vi "torreHanoi.vi"() -> ()   [LabVIEW 2020]
uses:
  <vilib>/Analysis/Matrix/Datatypes/RealMatrix.ctl
  <vilib>/Utility/miscctls.llb/LVPositionTypeDef.ctl
  <vilib>/Utility/miscctls.llb/LVBoundsTypeDef.ctl
  <vilib>/Analysis/Matrix/NI_Matrix.lvlib
panel:
  out "PosAntPiezaCuatro":T1
  out "PosAntPiezaCinco":T1
  out "PosAntPiezaTres":T1
  out "PosAntPiezaDos":T1
  out "Posicion":i32
  out "Torre":i8
  out "posPiezaDos":i32[][](array[numeric])
  out "posPiezaTres":i32[][](array[numeric])
  out "posPiezaUno":i32[][](array[numeric])
  out "posPiezaCinco":i32[](array[numeric])
  out "posPiezaCuatro":i32[][](array[numeric])
  out "estadoTorreTres":i32[](array[numeric])
  out "estadoTorreUno":i32[](array[numeric])
  out "estadoTorreDos":i32[](array[numeric])
  out "PosAntPiezaUno":T1
  out "¿Pieza?":i8
  out "matrizPosIniciales":T2
  out "numMov":dbl
  out "minMov":dbl
  in  "numPiezas":enum16{"5", "4", "3"}(ring)
  in  "Iniciar":bool
  out "PiezaCinco":bool
  out "PiezaCuatro":bool
  out "PiezaTres":bool
  out "PiezaDos":bool
  in  "Deterner":bool
  out "PiezaUno":bool
  out "TorreUno":u8(slide) scale=0.0..100.0
  out "TorreDos":u8(slide) scale=0.0..100.0
  out "TorreTres":u8(slide) scale=0.0..100.0
  # "Número de Piezas"
  # "Minimo de Movimientos"
  # "Tus Movimientos"
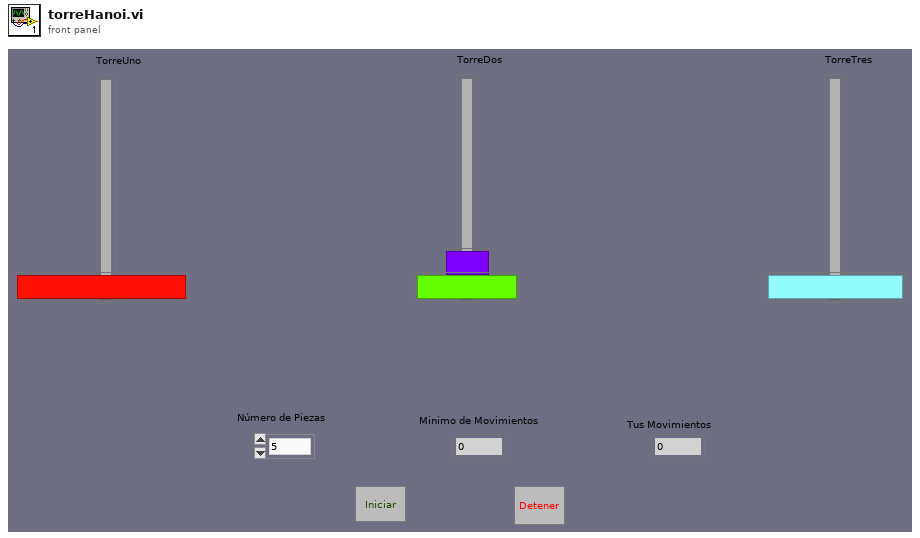
[diagram p1: front panel]
types:
  T1 = typedef "LVPositionTypeDef.ctl" = cluster{"Left":i32, "Top":i32}
  T2 = typedef "NI_Matrix.lvlib/RealMatrix.ctl" = dbl[][]
  T3 = typedef "LVBoundsTypeDef.ctl" = cluster{"Width":u32, "Height":u32}
  T4 = typedef "LVPoint32TypeDef.ctl" = cluster{"Horizontal":i32, "Vertical":i32}
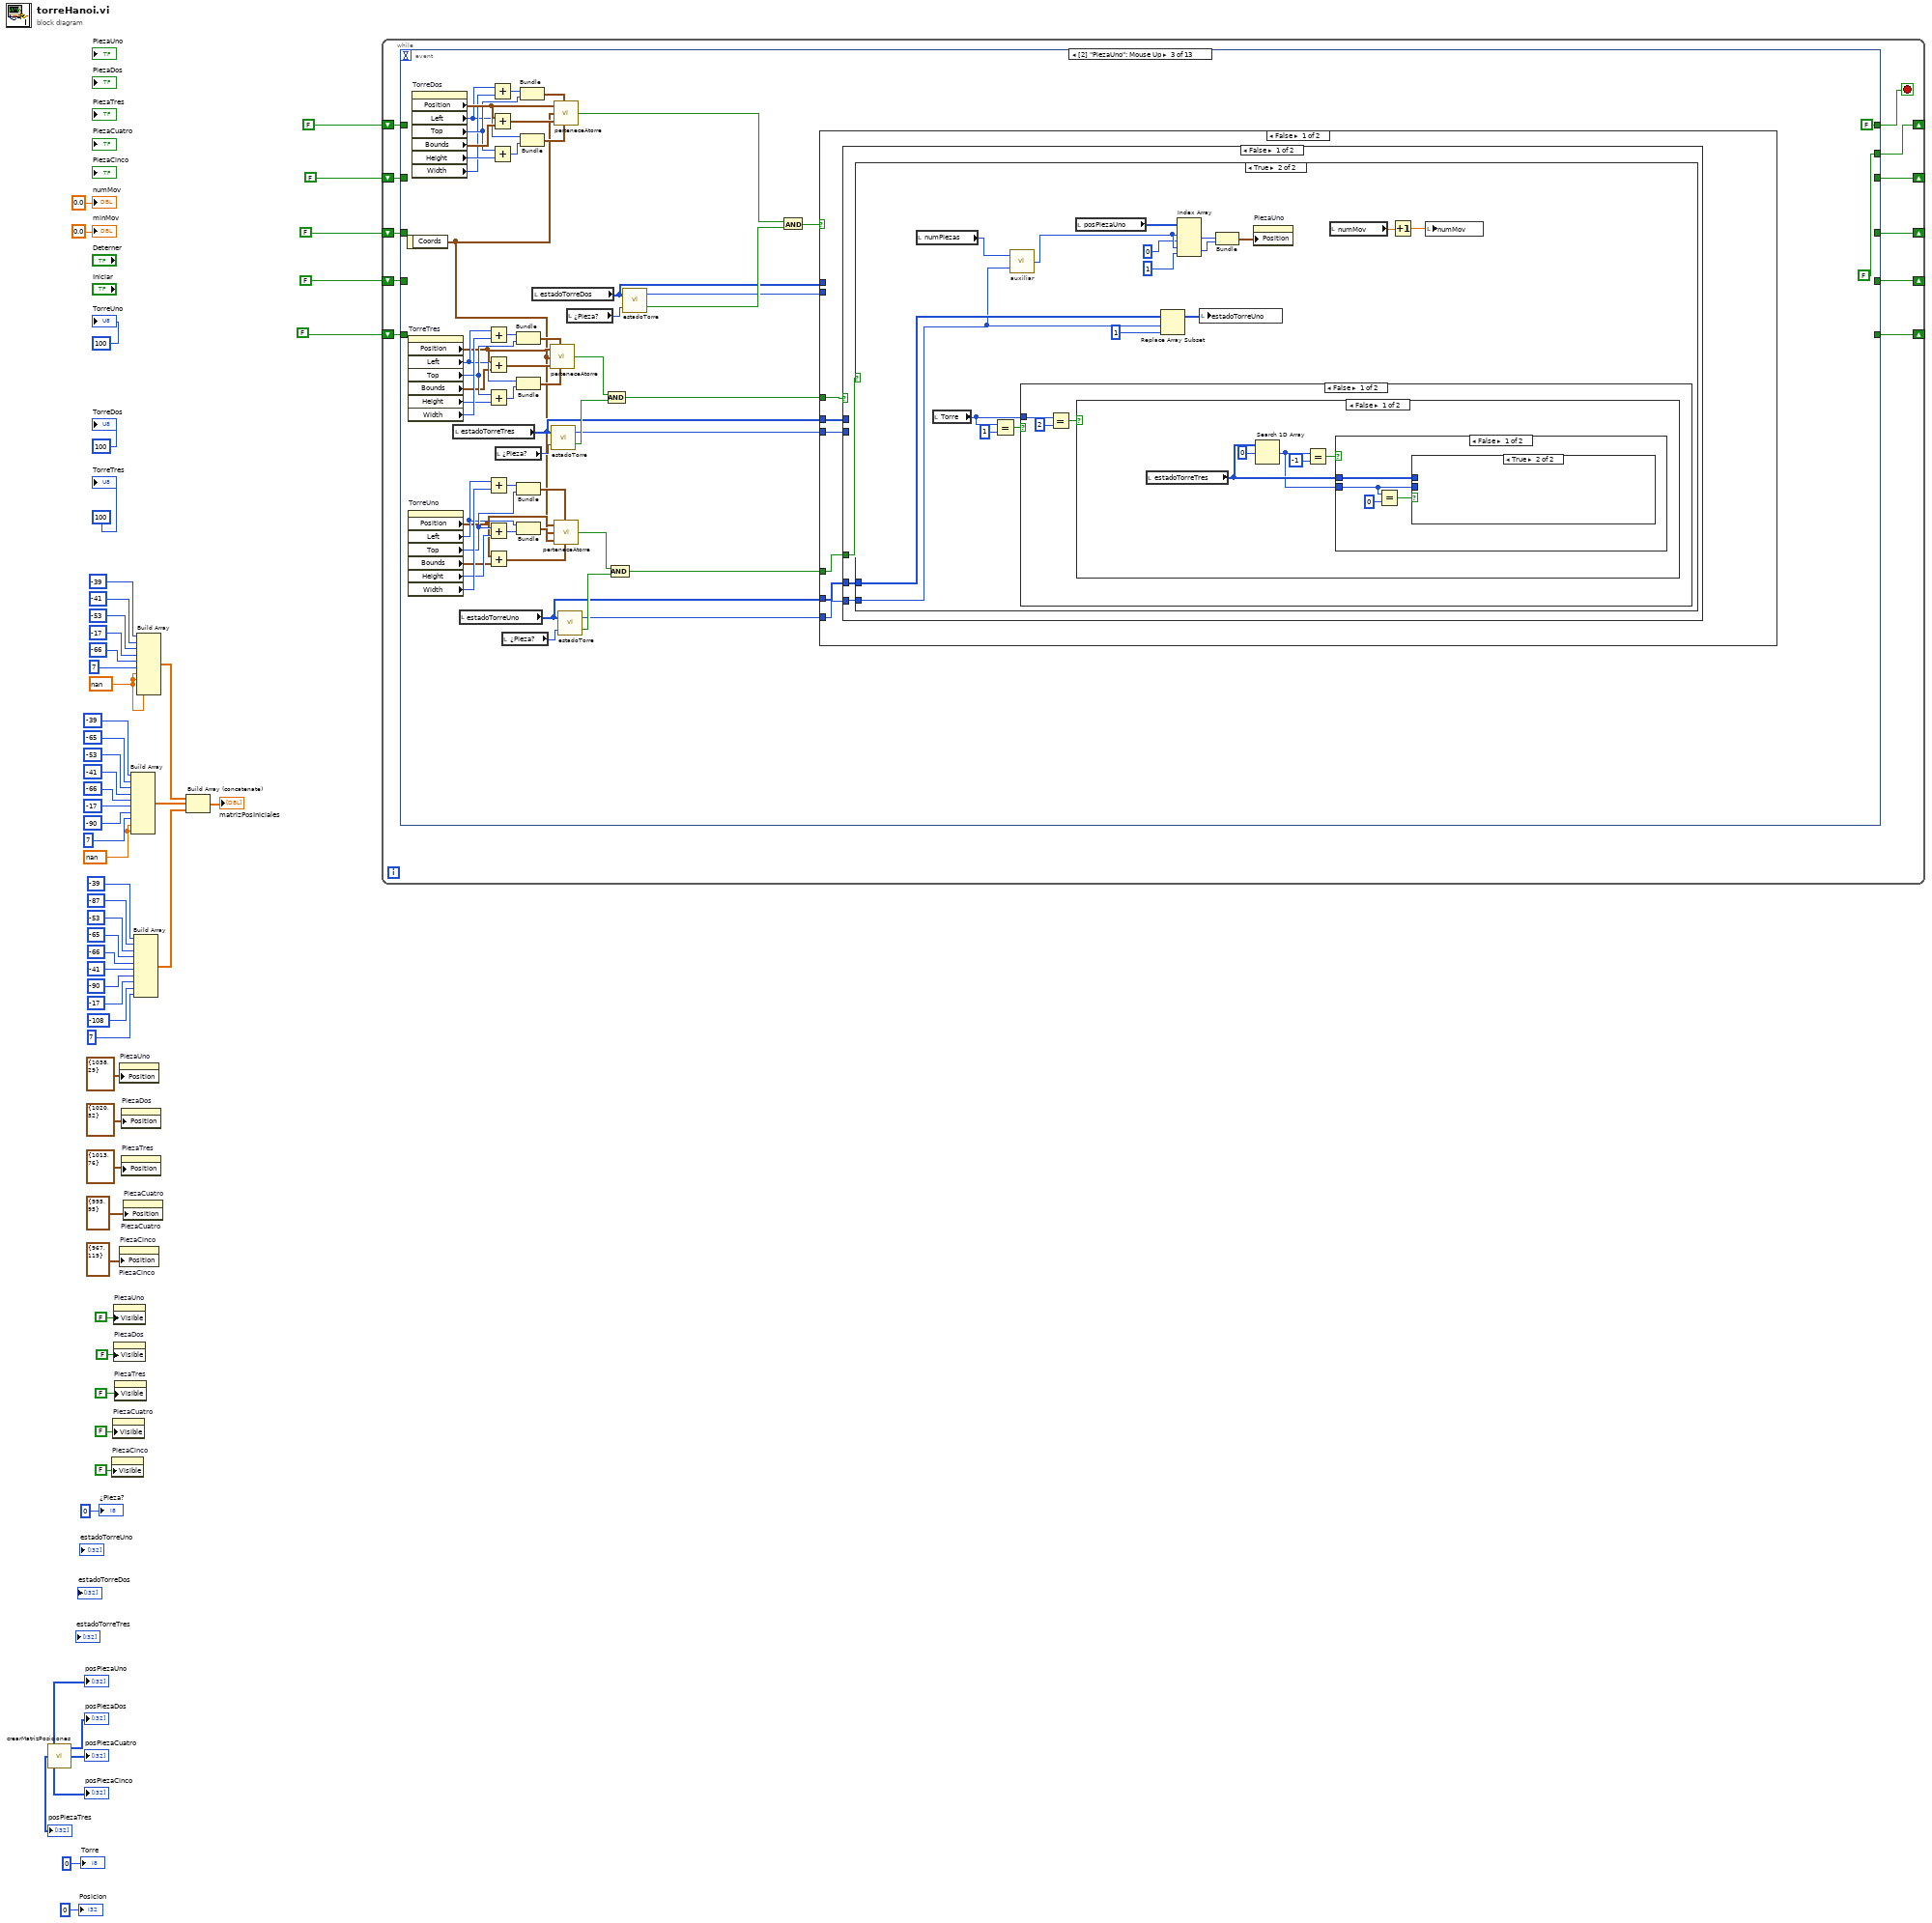
[diagram p0: block diagram]
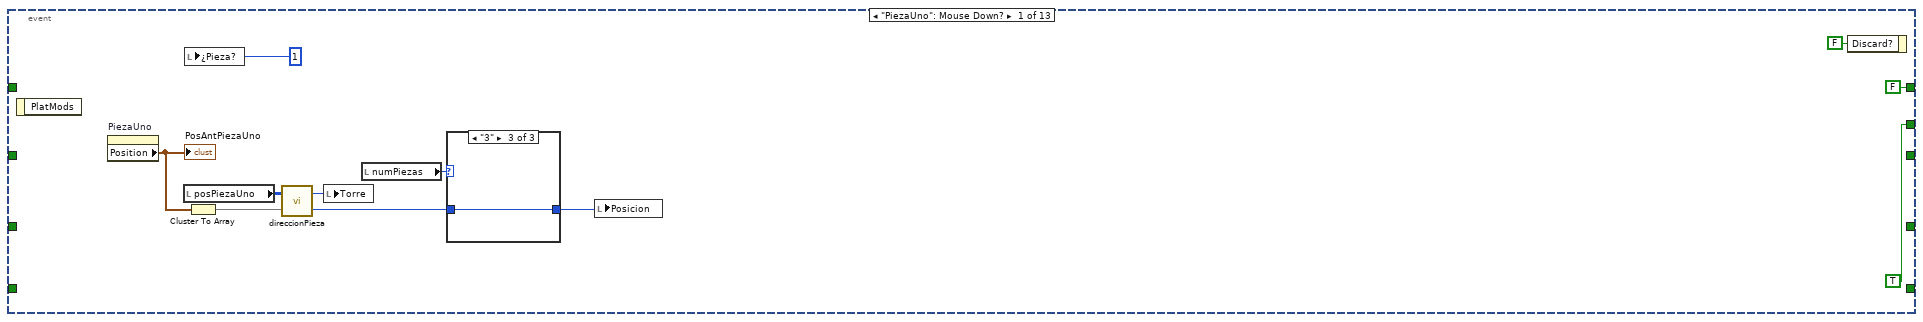
[diagram p2: hidden frame]
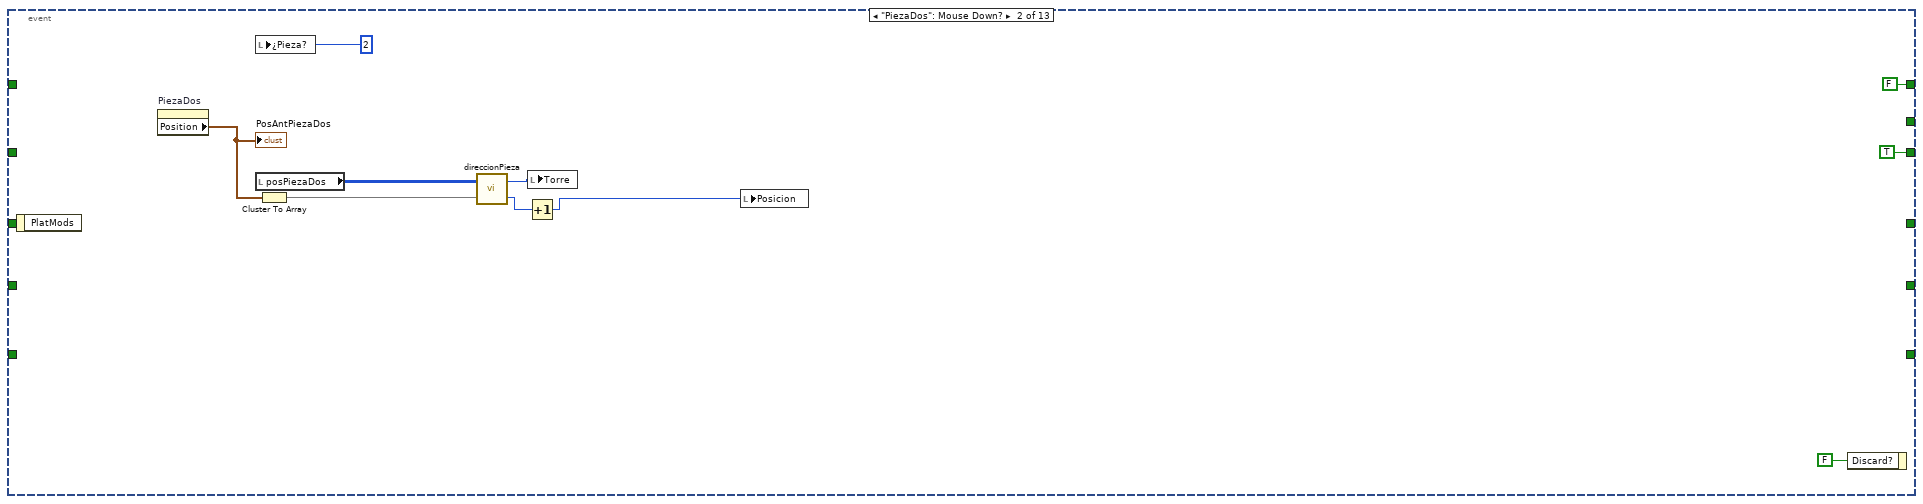
[diagram p5: hidden frame]
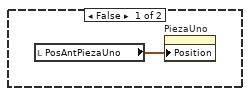
[diagram p6: hidden frame]
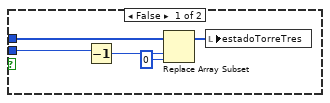
[diagram p7: hidden frame]
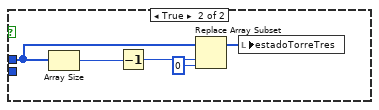
[diagram p8: hidden frame]
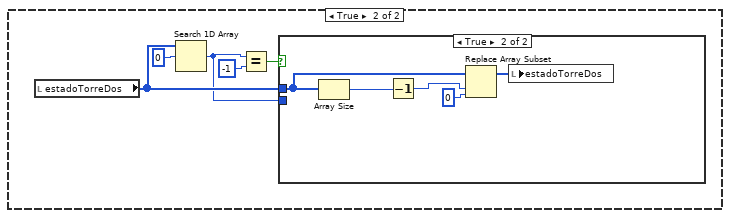
[diagram p9: hidden frame]
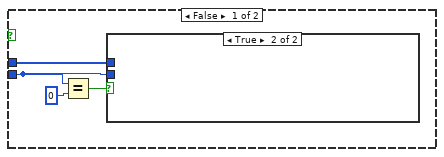
[diagram p10: hidden frame]
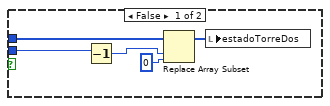
[diagram p11: hidden frame]
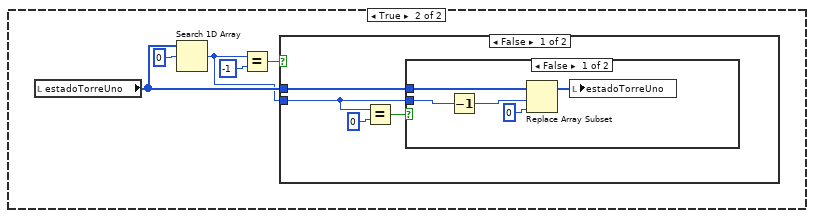
[diagram p12: hidden frame]
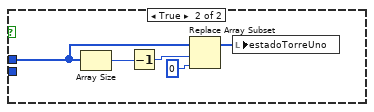
[diagram p14: hidden frame]
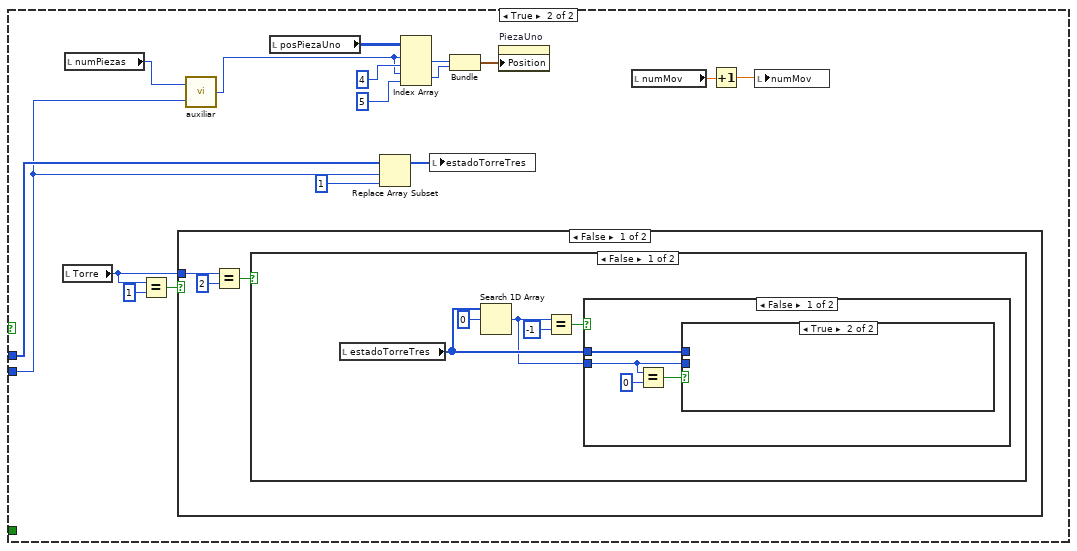
[diagram p15: hidden frame]
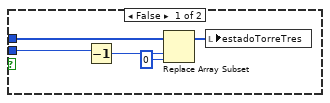
[diagram p16: hidden frame]
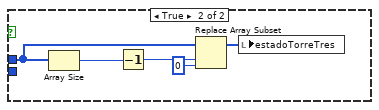
[diagram p17: hidden frame]
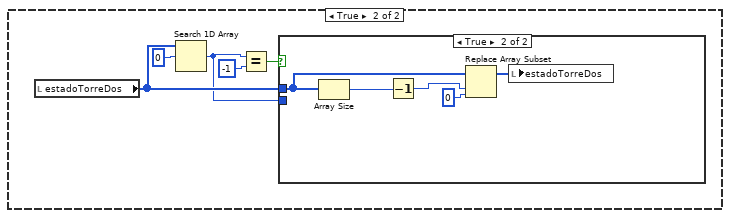
[diagram p18: hidden frame]
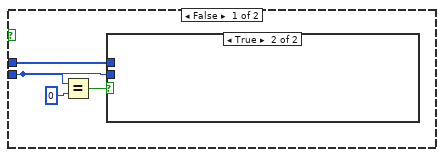
[diagram p19: hidden frame]
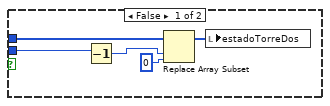
[diagram p20: hidden frame]
diagram:
  w42 = nan
  w51 = nan
  n1 = call "crearMatrizPosiciones.vi"() -> ("posPiezaCuatro"=→"posPiezaCuatro":i32[][], "posPiezaDos"=→"posPiezaDos":i32[][], "posPiezaCinco"=→"posPiezaCinco":i32[], "posPiezaTres"=→"posPiezaTres":i32[][], "posPiezaUno"=→"posPiezaUno":i32[][])  [unwired: 1 in]
  n2 = property on="PiezaCinco" class="Bool (strict)"("Visible"=FALSE ("PiezaCinco")) -> ()  [unwired: 2 in, 2 out]
  n3 = property on="PiezaCuatro" class="Bool (strict)"("Visible"=FALSE ("PiezaCuatro")) -> ()  [unwired: 2 in, 2 out]
  n4 = property on="PiezaUno" class="Bool (strict)"("Visible"=FALSE) -> ()  [unwired: 2 in, 2 out]
  n5 = property on="PiezaDos" class="Bool (strict)"("Visible"=FALSE ("PiezaDos")) -> ()  [unwired: 2 in, 2 out]
  n6 = property on="PiezaTres" class="Bool (strict)"("Visible"=FALSE) -> ()  [unwired: 2 in, 2 out]
  n7 = property on="PiezaUno" class="Bool (strict)"("Position"=T1 {"Left"=1038, "Top"=29}) -> ()  [unwired: 2 in, 2 out]
  n8 = property on="PiezaCinco" class="Bool (strict)"("Position"=T1 {"Left"=967, "Top"=119}) -> ()  [unwired: 2 in, 2 out]
  n9 = property on="PiezaCinco" class="Bool (strict)"("Position"=T1 {"Left"=967, "Top"=119}) -> ()  [unwired: 2 in, 2 out]
  n10 = property on="PiezaDos" class="Bool (strict)"("Position"=T1 {"Left"=1020, "Top"=52}) -> ()  [unwired: 2 in, 2 out]
  n11 = property on="PiezaTres" class="Bool (strict)"("Position"=T1 {"Left"=1013, "Top"=76}) -> ()  [unwired: 2 in, 2 out]
  n12 = property on="PiezaCuatro" class="Bool (strict)"("Position"=T1 {"Left"=995, "Top"=95}) -> ()  [unwired: 2 in, 2 out]
  n13 = property on="PiezaCuatro" class="Bool (strict)"("Position"=T1 {"Left"=995, "Top"=95}) -> ()  [unwired: 2 in, 2 out]
  n14 = Build Array(-39, -65 ("element"), -53 ("element"), -41 ("element"), -66 ("element"), -17 ("element"), -90 ("element"), 7 ("element"), w42, w42) -> (w30:T2)
  n15 = Build Array(-39, -87 ("element"), -53 ("element"), -65 ("element"), -66 ("element"), -41 ("element"), -90 ("element"), -17 ("element"), -108 ("element"), 7 ("element")) -> (w29:T2)
  n16 = Build Array(-39, -41 ("element"), -53 ("element"), -17 ("element"), -66 ("element"), 7 ("element"), w51, w51, w51, w51) -> (w31:T2)
  n17 = Build Array (concatenate)(w31, w30, w29) -> (→"matrizPosIniciales":T2)
  n18 = while {
    shift-right: [w70] -> _
    shift-left: FALSE -> [w69]
    shift-right: [w68] -> _
    shift-left: FALSE -> [w67]
    shift-right: [w66] -> _
    shift-left: FALSE -> [w65]
    shift-right: [w63] -> _
    shift-left: FALSE -> [w64]
    shift-right: [w62] -> _
    shift-left: FALSE -> [w61]
    stop <- w71 stop-if-true
    n19 = event shown="[2] \"PiezaUno\": Mouse Up" {
      selector: _ -> [_ _ _ _ _ _ _ _ _ _ _ _ _]
      dyn-events: _ -> [_ _ _ _ _ _ _ _ _ _ _ _ _]
      timeout: _ -> [_ _ _ _ _ _ _ _ _ _ _ _ _]
      tunnel: [FALSE FALSE FALSE FALSE FALSE TRUE _ FALSE FALSE FALSE FALSE FALSE _] -> w71
      tunnel: [TRUE _ FALSE w397 _ _ _ _ _ _ _ _ _] -> w70
      tunnel: w69 -> [_ _ _ w397 _ _ _ _ _ _ _ _ _]
      tunnel: [_ TRUE _ w395 _ _ _ FALSE _ _ _ _ _] -> w68
      tunnel: w67 -> [_ _ _ w395 _ _ _ _ _ _ _ _ _]
      tunnel: [_ _ _ w394 _ _ _ _ TRUE FALSE _ _ _] -> w66
      tunnel: w65 -> [_ _ _ w394 _ _ _ _ _ _ _ _ _]
      tunnel: w64 -> [_ _ _ w391 _ _ _ _ _ _ _ _ _]
      tunnel: [_ _ _ w391 FALSE _ _ _ _ _ TRUE _ _] -> w63
      tunnel: [_ _ _ w392 _ _ _ _ _ _ _ TRUE _] -> w62
      tunnel: w61 -> [_ _ _ w392 _ _ _ _ _ _ _ _ _]
      event "PiezaUno": Mouse Down? {
        n20 = event-data() -> ()  [unwired: 1 in, 1 out]
        n21 = property on="PiezaUno" class="Bool (strict)"() -> ("Position"=w78:T1)  [unwired: 2 in, 2 out]
        "PosAntPiezaUno" <- w78
        n22 = local read "posPiezaUno"() -> (w76:i32[][])
        n23 = local write "¿Pieza?"(i8 1 ("¿Pieza?")) -> ()
        n24 = Cluster To Array(cluster=w78) -> (array=w77:i32[])
        n25 = call "direccionPieza.vi"("posicion"=w77, "matrizPosiciones"=w76) -> ("Posicion"=w72:i32, "Torre"=w75:i8)
        n26 = local write "Torre"(w75) -> ()
        n27 = local read "numPiezas"() -> (w74:enum16{"5", "4", "3"})
        n28 = case shown="\"3\"" w74 {
          tunnel: [w83 w84 w85] -> w73
          tunnel: w72 -> [w83 w84 w85]
          frame "5", Default {
          }
          frame "4" {
          }
          frame "3" {
          }
        }
        n29 = local write "Posicion"(w73) -> ()
        n30 = event-data("Discard?"=FALSE) -> ()  [unwired: 1 in, 1 out]
      }
      event "PiezaDos": Mouse Down? {
        n31 = event-data() -> ()  [unwired: 1 in, 1 out]
        n32 = property on="PiezaDos" class="Bool (strict)"() -> ("Position"=w91:T1)  [unwired: 2 in, 2 out]
        "PosAntPiezaDos" <- w91
        n33 = local write "¿Pieza?"(i8 2 ("¿Pieza?")) -> ()
        n34 = local read "posPiezaDos"() -> (w93:i32[][])
        n35 = Cluster To Array(cluster=w91) -> (array=w94:i32[])
        n36 = call "direccionPieza.vi"("posicion"=w94, "matrizPosiciones"=w93) -> ("Posicion"=w87:i32, "Torre"=w92:i8)
        n37 = Increment(x=w87) -> (x+1=w86:i32)
        n38 = local write "Torre"(w92) -> ()
        n39 = local write "Posicion"(w86) -> ()
        n40 = event-data("Discard?"=FALSE) -> ()  [unwired: 1 in, 1 out]
      }
      event "PiezaUno": Mouse Up {
        n41 = event-data() -> ("Coords"=w102:T4)  [unwired: 1 in]
        n42 = property on="TorreTres" class="Slide (strict)"() -> ("Position"=w121:T1, "Left"=w124:i32, "Top"=w127:i32, "Bounds"=w122:T3, "Height"=w126:u32, "Width"=w130:u32)  [unwired: 2 in, 2 out]
        n43 = property on="TorreUno" class="Slide (strict)"() -> ("Position"=w105:T1, "Left"=w107:i32, "Top"=w110:i32, "Bounds"=w104:T3, "Height"=w109:u32, "Width"=w113:u32)  [unwired: 2 in, 2 out]
        n44 = property on="TorreDos" class="Slide (strict)"() -> ("Position"=w144:T1, "Left"=w139:i32, "Top"=w142:i32, "Bounds"=w145:T3, "Height"=w141:u32, "Width"=w140:u32)  [unwired: 2 in, 2 out]
        n45 = local read "estadoTorreTres"() -> (w115:i32[])
        n46 = local read "estadoTorreUno"() -> (w96:i32[])
        n47 = Add(x=w124, y=w130) -> (x+y=w129:u32)
        n48 = Add(x=w121, y=w122) -> (x+y=w120:T3)
        n49 = Add(x=w127, y=w126) -> (x+y=w125:u32)
        n50 = Add(x=w107, y=w113) -> (x+y=w111:u32)
        n51 = Add(x=w110, y=w109) -> (x+y=w108:u32)
        n52 = Add(x=w105, y=w104) -> (x+y=w103:T3)
        n53 = Add(x=w139, y=w140) -> (x+y=w147:u32)
        n54 = Add(x=w144, y=w145) -> (x+y=w143:T3)
        n55 = Add(x=w142, y=w141) -> (x+y=w138:u32)
        n56 = local read "¿Pieza?"() -> (w119:i8)
        n57 = local read "¿Pieza?"() -> (w101:i8)
        n58 = Bundle(w129, "Top"=w127) -> (w128:cluster{u32, "Top":i32})  [unwired: 1 in]
        n59 = Bundle("Left"=w124, w125) -> (w123:cluster{"Left":i32, u32})  [unwired: 1 in]
        n60 = Bundle(w111, "Top"=w110) -> (w112:cluster{u32, "Top":i32})  [unwired: 1 in]
        n61 = Bundle("Left"=w107, w108) -> (w106:cluster{"Left":i32, u32})  [unwired: 1 in]
        n62 = Bundle(w147, "Top"=w142) -> (w146:cluster{u32, "Top":i32})  [unwired: 1 in]
        n63 = Bundle("Left"=w139, w138) -> (w137:cluster{"Left":i32, u32})  [unwired: 1 in]
        n64 = local read "estadoTorreDos"() -> (w131:i32[])
        n65 = call "perteneceAtorre.vi"("P1"=w121, "P2"=w128, "P"=w102, "P3"=w120, "P4"=w123) -> ("out"=w118:bool)
        n66 = call "estadoTorre.vi"("¿pieza?"=w119, "estadoTorre"=w115) -> ("¿disponible?"=w117:bool, "posicionCero"=w116:i32)
        n67 = call "perteneceAtorre.vi"("P1"=w144, "P2"=w146, "P"=w102, "P3"=w143, "P4"=w137) -> ("out"=w135:bool)
        n68 = call "perteneceAtorre.vi"("P1"=w105, "P2"=w112, "P"=w102, "P3"=w106, "P4"=w103) -> ("out"=w100:bool)
        n69 = call "estadoTorre.vi"("¿pieza?"=w101, "estadoTorre"=w96) -> ("¿disponible?"=w99:bool, "posicionCero"=w97:i32)
        n70 = local read "¿Pieza?"() -> (w134:i8)
        n71 = And(x=w118, y=w117) -> (x .and. y?=w114:bool)
        n72 = And(x=w100, y=w99) -> (x .and. y?=w98:bool)
        n73 = call "estadoTorre.vi"("¿pieza?"=w134, "estadoTorre"=w131) -> ("¿disponible?"=w133:bool, "posicionCero"=w132:i32)
        n74 = And(x=w135, y=w133) -> (x .and. y?=w136:bool)
        n75 = case shown="False" w136 {
          tunnel: w132 -> [_ w320]
          tunnel: w131 -> [_ w324]
          tunnel: w116 -> [w153 _]
          tunnel: w115 -> [w154 _]
          tunnel: w114 -> [w155 _]
          tunnel: w98 -> [w152 _]
          tunnel: w97 -> [w150 _]
          tunnel: w96 -> [w151 _]
          frame False {
            n76 = case shown="False" w155 {
              tunnel: w154 -> [_ w243]
              tunnel: w153 -> [_ w242]
              tunnel: w152 -> [w158 _]
              tunnel: w151 -> [w157 _]
              tunnel: w150 -> [w156 _]
              frame False {
                n77 = case shown="True" w158 {
                  tunnel: w157 -> [_ w166]
                  tunnel: w156 -> [_ w165]
                  frame False {
                    n78 = local read "PosAntPiezaUno"() -> (w159:T1)
                    n79 = property on="PiezaUno" class="Bool (strict)"("Position"=w159) -> ()  [unwired: 2 in, 2 out]
                  }
                  frame True {
                    n80 = local read "numPiezas"() -> (w171:enum16{"5", "4", "3"})
                    n81 = local read "Torre"() -> (w160:i8)
                    n82 = Equal?(x=w160, y=i8 1) -> (x = y?=w162:bool)
                    n83 = call "auxiliar.vi"("posicion"=w165, "numPiezas"=w171) -> ("posicion"=w170:i32)
                    n84 = case shown="False" w162 {
                      tunnel: w160 -> [w177 _]
                      frame False {
                        n85 = Equal?(x=w177, y=i8 2) -> (x = y?=w178:bool)
                        n86 = case shown="False" w178 {
                          frame False {
                            n87 = local read "estadoTorreTres"() -> (w183:i32[])
                            n88 = Search 1D Array(1D array=w183, element=0) -> (index of element=w182:i32)  [unwired: 1 in]
                            n89 = Equal?(x=w182, y=-1) -> (x = y?=w184:bool)
                            n90 = case shown="False" w184 {
                              tunnel: w183 -> [w185 w196]
                              tunnel: w182 -> [w186 _]
                              frame False {
                                n91 = Equal?(x=w186, y=0) -> (x = y?=w187:bool)
                                n92 = case shown="True" w187 {
                                tunnel: w186 -> [w193 _]
                                tunnel: w185 -> [w191 _]
                                frame False {
                                n93 = Decrement(x=w193) -> (x-1=w192:i32)
                                n94 = Replace Array Subset(array=w191, new element=0 ("new element/subarray"), index=w192) -> (w189:i32[])
                                n95 = local write "estadoTorreTres"(w189) -> ()
                                }
                                frame True {
                                }
                                }
                              }
                              frame True {
                                n96 = Array Size(array=w196) -> (size(s)=w198:i32)
                                n97 = Decrement(x=w198) -> (x-1=w197:i32)
                                n98 = Replace Array Subset(array=w196, new element=0 ("new element/subarray"), index=w197) -> (w194:i32[])
                                n99 = local write "estadoTorreTres"(w194) -> ()
                              }
                            }
                          }
                          frame True {
                            n100 = local read "estadoTorreDos"() -> (w200:i32[])
                            n101 = Search 1D Array(1D array=w200, element=0) -> (index of element=w199:i32)  [unwired: 1 in]
                            n102 = Equal?(x=w199, y=-1) -> (x = y?=w201:bool)
                            n103 = case shown="True" w201 {
                              tunnel: w200 -> [w204 w215]
                              tunnel: w199 -> [w205 _]
                              frame False {
                                n104 = Equal?(x=w205, y=0) -> (x = y?=w206:bool)
                                n105 = case shown="True" w206 {
                                tunnel: w205 -> [w212 _]
                                tunnel: w204 -> [w210 _]
                                frame False {
                                n106 = Decrement(x=w212) -> (x-1=w211:i32)
                                n107 = Replace Array Subset(array=w210, new element=0 ("new element/subarray"), index=w211) -> (w208:i32[])
                                n108 = local write "estadoTorreDos"(w208) -> ()
                                }
                                frame True {
                                }
                                }
                              }
                              frame True {
                                n109 = Array Size(array=w215) -> (size(s)=w217:i32)
                                n110 = Decrement(x=w217) -> (x-1=w216:i32)
                                n111 = Replace Array Subset(array=w215, new element=0 ("new element/subarray"), index=w216) -> (w213:i32[])
                                n112 = local write "estadoTorreDos"(w213) -> ()
                              }
                            }
                          }
                        }
                      }
                      frame True {
                        n113 = local read "estadoTorreUno"() -> (w219:i32[])
                        n114 = Search 1D Array(1D array=w219, element=0) -> (index of element=w218:i32)  [unwired: 1 in]
                        n115 = Equal?(x=w218, y=-1) -> (x = y?=w220:bool)
                        n116 = case shown="False" w220 {
                          tunnel: w219 -> [w223 w234]
                          tunnel: w218 -> [w224 _]
                          frame False {
                            n117 = Equal?(x=w224, y=0) -> (x = y?=w225:bool)
                            n118 = case shown="False" w225 {
                              tunnel: w224 -> [w231 _]
                              tunnel: w223 -> [w229 _]
                              frame False {
                                n119 = Decrement(x=w231) -> (x-1=w230:i32)
                                n120 = Replace Array Subset(array=w229, new element=0 ("new element/subarray"), index=w230) -> (w227:i32[])
                                n121 = local write "estadoTorreUno"(w227) -> ()
                              }
                              frame True {
                              }
                            }
                          }
                          frame True {
                            n122 = Array Size(array=w234) -> (size(s)=w236:i32)
                            n123 = Decrement(x=w236) -> (x-1=w235:i32)
                            n124 = Replace Array Subset(array=w234, new element=0 ("new element/subarray"), index=w235) -> (w232:i32[])
                            n125 = local write "estadoTorreUno"(w232) -> ()
                          }
                        }
                      }
                    }
                    n126 = local read "posPiezaUno"() -> (w175:i32[][])
                    n127 = Replace Array Subset(array=w166, new element=1, index=w165) -> (w176:i32[])
                    n128 = Index Array(array=w175, index (row) #1=w170, index (col) #1=0 ("disabled index (col)"), index (row) #2=w170, index (col) #2=1 ("disabled index (col)")) -> (element #1=w174:i32, element #2=w172:i32)
                    n129 = local write "estadoTorreUno"(w176) -> ()
                    n130 = Bundle(w174, w172) -> (w173:cluster{i32, i32})  [unwired: 1 in]
                    n131 = property on="PiezaUno" class="Bool (strict)"("Position"=w173) -> ()  [unwired: 2 in, 2 out]
                    n132 = local read "numMov"() -> (w164:dbl)
                    n133 = Increment(x=w164) -> (x+1=w163:dbl)
                    n134 = local write "numMov"(w163) -> ()
                  }
                }
              }
              frame True {
                n135 = local read "Torre"() -> (w238:i8)
                n136 = local read "numPiezas"() -> (w245:enum16{"5", "4", "3"})
                n137 = Equal?(x=w238, y=i8 1) -> (x = y?=w239:bool)
                n138 = case shown="False" w239 {
                  tunnel: w238 -> [w254 _]
                  frame False {
                    n139 = Equal?(x=w254, y=i8 2) -> (x = y?=w255:bool)
                    n140 = case shown="False" w255 {
                      frame False {
                        n141 = local read "estadoTorreTres"() -> (w260:i32[])
                        n142 = Search 1D Array(1D array=w260, element=0) -> (index of element=w259:i32)  [unwired: 1 in]
                        n143 = Equal?(x=w259, y=-1) -> (x = y?=w261:bool)
                        n144 = case shown="False" w261 {
                          tunnel: w260 -> [w262 w273]
                          tunnel: w259 -> [w263 _]
                          frame False {
                            n145 = Equal?(x=w263, y=0) -> (x = y?=w264:bool)
                            n146 = case shown="True" w264 {
                              tunnel: w263 -> [w270 _]
                              tunnel: w262 -> [w268 _]
                              frame False {
                                n147 = Decrement(x=w270) -> (x-1=w269:i32)
                                n148 = Replace Array Subset(array=w268, new element=0 ("new element/subarray"), index=w269) -> (w266:i32[])
                                n149 = local write "estadoTorreTres"(w266) -> ()
                              }
                              frame True {
                              }
                            }
                          }
                          frame True {
                            n150 = Array Size(array=w273) -> (size(s)=w275:i32)
                            n151 = Decrement(x=w275) -> (x-1=w274:i32)
                            n152 = Replace Array Subset(array=w273, new element=0 ("new element/subarray"), index=w274) -> (w271:i32[])
                            n153 = local write "estadoTorreTres"(w271) -> ()
                          }
                        }
                      }
                      frame True {
                        n154 = local read "estadoTorreDos"() -> (w277:i32[])
                        n155 = Search 1D Array(1D array=w277, element=0) -> (index of element=w276:i32)  [unwired: 1 in]
                        n156 = Equal?(x=w276, y=-1) -> (x = y?=w278:bool)
                        n157 = case shown="True" w278 {
                          tunnel: w277 -> [w281 w292]
                          tunnel: w276 -> [w282 _]
                          frame False {
                            n158 = Equal?(x=w282, y=0) -> (x = y?=w283:bool)
                            n159 = case shown="True" w283 {
                              tunnel: w282 -> [w289 _]
                              tunnel: w281 -> [w287 _]
                              frame False {
                                n160 = Decrement(x=w289) -> (x-1=w288:i32)
                                n161 = Replace Array Subset(array=w287, new element=0 ("new element/subarray"), index=w288) -> (w285:i32[])
                                n162 = local write "estadoTorreDos"(w285) -> ()
                              }
                              frame True {
                              }
                            }
                          }
                          frame True {
                            n163 = Array Size(array=w292) -> (size(s)=w294:i32)
                            n164 = Decrement(x=w294) -> (x-1=w293:i32)
                            n165 = Replace Array Subset(array=w292, new element=0 ("new element/subarray"), index=w293) -> (w290:i32[])
                            n166 = local write "estadoTorreDos"(w290) -> ()
                          }
                        }
                      }
                    }
                  }
                  frame True {
                    n167 = local read "estadoTorreUno"() -> (w296:i32[])
                    n168 = Search 1D Array(1D array=w296, element=0) -> (index of element=w295:i32)  [unwired: 1 in]
                    n169 = Equal?(x=w295, y=-1) -> (x = y?=w297:bool)
                    n170 = case shown="False" w297 {
                      tunnel: w296 -> [w300 w311]
                      tunnel: w295 -> [w301 _]
                      frame False {
                        n171 = Equal?(x=w301, y=0) -> (x = y?=w302:bool)
                        n172 = case shown="False" w302 {
                          tunnel: w301 -> [w308 _]
                          tunnel: w300 -> [w306 _]
                          frame False {
                            n173 = Decrement(x=w308) -> (x-1=w307:i32)
                            n174 = Replace Array Subset(array=w306, new element=0 ("new element/subarray"), index=w307) -> (w304:i32[])
                            n175 = local write "estadoTorreUno"(w304) -> ()
                          }
                          frame True {
                          }
                        }
                      }
                      frame True {
                        n176 = Array Size(array=w311) -> (size(s)=w313:i32)
                        n177 = Decrement(x=w313) -> (x-1=w312:i32)
                        n178 = Replace Array Subset(array=w311, new element=0 ("new element/subarray"), index=w312) -> (w309:i32[])
                        n179 = local write "estadoTorreUno"(w309) -> ()
                      }
                    }
                  }
                }
                n180 = call "auxiliar.vi"("posicion"=w242, "numPiezas"=w245) -> ("posicion"=w244:i32)
                n181 = local read "posPiezaUno"() -> (w251:i32[][])
                n182 = Replace Array Subset(array=w243, new element=1, index=w242) -> (w252:i32[])
                n183 = Index Array(array=w251, index (row) #1=w244, index (col) #1=4 ("disabled index (col)"), index (row) #2=w244, index (col) #2=5 ("disabled index (col)")) -> (element #1=w248:i32, element #2=w246:i32)
                n184 = local write "estadoTorreTres"(w252) -> ()
                n185 = Bundle(w248, w246) -> (w247:cluster{i32, i32})  [unwired: 1 in]
                n186 = property on="PiezaUno" class="Bool (strict)"("Position"=w247) -> ()  [unwired: 2 in, 2 out]
                n187 = local read "numMov"() -> (w241:dbl)
                n188 = Increment(x=w241) -> (x+1=w240:dbl)
                n189 = local write "numMov"(w240) -> ()
              }
            }
          }
          frame True {
            n190 = local read "numPiezas"() -> (w321:enum16{"5", "4", "3"})
            n191 = local read "Torre"() -> (w314:i8)
            n192 = call "auxiliar.vi"("posicion"=w320, "numPiezas"=w321) -> ("posicion"=w319:i32)
            n193 = Equal?(x=w314, y=i8 1) -> (x = y?=w316:bool)
            n194 = case shown="False" w316 {
              tunnel: w314 -> [w331 _]
              frame False {
                n195 = Equal?(x=w331, y=i8 2) -> (x = y?=w332:bool)
                n196 = case shown="False" w332 {
                  frame False {
                    n197 = local read "estadoTorreTres"() -> (w337:i32[])
                    n198 = Search 1D Array(1D array=w337, element=0) -> (index of element=w336:i32)  [unwired: 1 in]
                    n199 = Equal?(x=w336, y=-1) -> (x = y?=w338:bool)
                    n200 = case shown="False" w338 {
                      tunnel: w337 -> [w339 w350]
                      tunnel: w336 -> [w340 _]
                      frame False {
                        n201 = Equal?(x=w340, y=0) -> (x = y?=w341:bool)
                        n202 = case shown="True" w341 {
                          tunnel: w340 -> [w347 _]
                          tunnel: w339 -> [w345 _]
                          frame False {
                            n203 = Decrement(x=w347) -> (x-1=w346:i32)
                            n204 = Replace Array Subset(array=w345, new element=0 ("new element/subarray"), index=w346) -> (w343:i32[])
                            n205 = local write "estadoTorreTres"(w343) -> ()
                          }
                          frame True {
                          }
                        }
                      }
                      frame True {
                        n206 = Array Size(array=w350) -> (size(s)=w352:i32)
                        n207 = Decrement(x=w352) -> (x-1=w351:i32)
                        n208 = Replace Array Subset(array=w350, new element=0 ("new element/subarray"), index=w351) -> (w348:i32[])
                        n209 = local write "estadoTorreTres"(w348) -> ()
                      }
                    }
                  }
                  frame True {
                    n210 = local read "estadoTorreDos"() -> (w354:i32[])
                    n211 = Search 1D Array(1D array=w354, element=0) -> (index of element=w353:i32)  [unwired: 1 in]
                    n212 = Equal?(x=w353, y=-1) -> (x = y?=w355:bool)
                    n213 = case shown="True" w355 {
                      tunnel: w354 -> [w358 w369]
                      tunnel: w353 -> [w359 _]
                      frame False {
                        n214 = Equal?(x=w359, y=0) -> (x = y?=w360:bool)
                        n215 = case shown="True" w360 {
                          tunnel: w359 -> [w366 _]
                          tunnel: w358 -> [w364 _]
                          frame False {
                            n216 = Decrement(x=w366) -> (x-1=w365:i32)
                            n217 = Replace Array Subset(array=w364, new element=0 ("new element/subarray"), index=w365) -> (w362:i32[])
                            n218 = local write "estadoTorreDos"(w362) -> ()
                          }
                          frame True {
                          }
                        }
                      }
                      frame True {
                        n219 = Array Size(array=w369) -> (size(s)=w371:i32)
                        n220 = Decrement(x=w371) -> (x-1=w370:i32)
                        n221 = Replace Array Subset(array=w369, new element=0 ("new element/subarray"), index=w370) -> (w367:i32[])
                        n222 = local write "estadoTorreDos"(w367) -> ()
                      }
                    }
                  }
                }
              }
              frame True {
                n223 = local read "estadoTorreUno"() -> (w373:i32[])
                n224 = Search 1D Array(1D array=w373, element=0) -> (index of element=w372:i32)  [unwired: 1 in]
                n225 = Equal?(x=w372, y=-1) -> (x = y?=w374:bool)
                n226 = case shown="False" w374 {
                  tunnel: w373 -> [w377 w388]
                  tunnel: w372 -> [w378 _]
                  frame False {
                    n227 = Equal?(x=w378, y=0) -> (x = y?=w379:bool)
                    n228 = case shown="False" w379 {
                      tunnel: w378 -> [w385 _]
                      tunnel: w377 -> [w383 _]
                      frame False {
                        n229 = Decrement(x=w385) -> (x-1=w384:i32)
                        n230 = Replace Array Subset(array=w383, new element=0 ("new element/subarray"), index=w384) -> (w381:i32[])
                        n231 = local write "estadoTorreUno"(w381) -> ()
                      }
                      frame True {
                      }
                    }
                  }
                  frame True {
                    n232 = Array Size(array=w388) -> (size(s)=w390:i32)
                    n233 = Decrement(x=w390) -> (x-1=w389:i32)
                    n234 = Replace Array Subset(array=w388, new element=0 ("new element/subarray"), index=w389) -> (w386:i32[])
                    n235 = local write "estadoTorreUno"(w386) -> ()
                  }
                }
              }
            }
            n236 = local read "posPiezaUno"() -> (w328:i32[][])
            n237 = Replace Array Subset(array=w324, new element=1, index=w320) -> (w329:i32[])
            n238 = Index Array(array=w328, index (row) #1=w319, index (col) #1=2 ("disabled index (col)"), index (row) #2=w319, index (col) #2=3 ("disabled index (col)")) -> (element #1=w325:i32, element #2=w322:i32)
            n239 = local write "estadoTorreDos"(w329) -> ()
            n240 = Bundle(w325, w322) -> (w323:cluster{i32, i32})  [unwired: 1 in]
            n241 = property on="PiezaUno" class="Bool (strict)"("Position"=w323) -> ()  [unwired: 2 in, 2 out]
            n242 = local read "numMov"() -> (w318:dbl)
            n243 = Increment(x=w318) -> (x+1=w317:dbl)
            n244 = local write "numMov"(w317) -> ()
          }
        }
      }
      event Mouse Move {
        n245 = event-data() -> ("Coords"=w393:T4)  [unwired: 1 in]
        n246 = case shown="True" w394 {
          tunnel: w393 -> [_ w410]
          frame False {
          }
          frame True {
            n247 = property on="PiezaTres" class="Bool (strict)"() -> ("Bounds"=w409:T3)  [unwired: 2 in, 2 out]
            n248 = Divide(x=w409, y=T3 {"Width"=2, "Height"=2}) -> (x/y=w411:cluster{"Width":dbl, "Height":dbl})
            n249 = Subtract(x=w410, y=w411) -> (x-y=w408:cluster{dbl, dbl})
            n250 = property on="PiezaTres" class="Bool (strict)"("Position"=w408) -> ()  [unwired: 2 in, 2 out]
          }
        }
        n251 = case shown="True" w395 {
          tunnel: w393 -> [_ w415]
          frame False {
          }
          frame True {
            n252 = property on="PiezaDos" class="Bool (strict)"() -> ("Bounds"=w414:T3)  [unwired: 2 in, 2 out]
            n253 = Divide(x=w414, y=T3 {"Width"=2, "Height"=2}) -> (x/y=w416:cluster{"Width":dbl, "Height":dbl})
            n254 = Subtract(x=w415, y=w416) -> (x-y=w413:cluster{dbl, dbl})
            n255 = property on="PiezaDos" class="Bool (strict)"("Position"=w413) -> ()  [unwired: 2 in, 2 out]
          }
        }
        n256 = case shown="True" w397 {
          tunnel: w393 -> [_ w419]
          frame False {
          }
          frame True {
            n257 = property on="PiezaUno" class="Bool (strict)"() -> ("Bounds"=w422:T3)  [unwired: 2 in, 2 out]
            n258 = Divide(x=w422, y=T3 {"Width"=2, "Height"=2}) -> (x/y=w420:cluster{"Width":dbl, "Height":dbl})
            n259 = Subtract(x=w419, y=w420) -> (x-y=w418:cluster{dbl, dbl})
            n260 = property on="PiezaUno" class="Bool (strict)"("Position"=w418) -> ()  [unwired: 2 in, 2 out]
          }
        }
        n261 = case shown="True" w391 {
          tunnel: w393 -> [_ w405]
          frame False {
          }
          frame True {
            n262 = property on="PiezaCuatro" class="Bool (strict)"() -> ("Bounds"=w403:T3)  [unwired: 2 in, 2 out]
            n263 = Divide(x=w403, y=T3 {"Width"=2, "Height"=2}) -> (x/y=w406:cluster{"Width":dbl, "Height":dbl})
            n264 = Subtract(x=w405, y=w406) -> (x-y=w404:cluster{dbl, dbl})
            n265 = property on="PiezaCuatro" class="Bool (strict)"("Position"=w404) -> ()  [unwired: 2 in, 2 out]
          }
        }
        n266 = case shown="True" w392 {
          tunnel: w393 -> [_ w400]
          frame False {
          }
          frame True {
            n267 = property on="PiezaCinco" class="Bool (strict)"() -> ("Bounds"=w399:T3)  [unwired: 2 in, 2 out]
            n268 = Divide(x=w399, y=T3 {"Width"=2, "Height"=2}) -> (x/y=w401:cluster{"Width":dbl, "Height":dbl})
            n269 = Subtract(x=w400, y=w401) -> (x-y=w398:cluster{dbl, dbl})
            n270 = property on="PiezaCinco" class="Bool (strict)"("Position"=w398) -> ()  [unwired: 2 in, 2 out]
          }
        }
      }
      event "PiezaCuatro": Mouse Up {
        n271 = event-data() -> ("Coords"=w474:T4)  [unwired: 1 in]
        n272 = property on="TorreUno" class="Slide (strict)"() -> ("Position"=w438:T1, "Left"=w440:i32, "Top"=w443:i32, "Bounds"=w437:T3, "Height"=w442:u32, "Width"=w432:u32)  [unwired: 2 in, 2 out]
        n273 = property on="TorreTres" class="Slide (strict)"() -> ("Position"=w447:T1, "Left"=w450:i32, "Top"=w453:i32, "Bounds"=w448:T3, "Height"=w452:u32, "Width"=w456:u32)  [unwired: 2 in, 2 out]
        n274 = property on="TorreDos" class="Slide (strict)"() -> ("Position"=w462:T1, "Left"=w458:i32, "Top"=w460:i32, "Bounds"=w463:T3, "Height"=w459:u32, "Width"=w434:u32)  [unwired: 2 in, 2 out]
        n275 = local read "estadoTorreTres"() -> (w469:i32[])
        n276 = local read "estadoTorreDos"() -> (w472:i32[])
        n277 = local read "estadoTorreUno"() -> (w466:i32[])
        n278 = local read "¿Pieza?"() -> (w430:i8)
        n279 = local read "¿Pieza?"() -> (w431:i8)
        n280 = local read "¿Pieza?"() -> (w429:i8)
        n281 = Add(x=w440, y=w432) -> (x+y=w444:u32)
        n282 = Add(x=w443, y=w442) -> (x+y=w441:u32)
        n283 = Add(x=w438, y=w437) -> (x+y=w436:T3)
        n284 = Add(x=w450, y=w456) -> (x+y=w455:u32)
        n285 = Add(x=w447, y=w448) -> (x+y=w446:T3)
        n286 = Add(x=w453, y=w452) -> (x+y=w451:u32)
        n287 = Add(x=w458, y=w434) -> (x+y=w464:u32)
        n288 = Add(x=w462, y=w463) -> (x+y=w461:T3)
        n289 = Add(x=w460, y=w459) -> (x+y=w457:u32)
        n290 = call "estadoTorre.vi"("¿pieza?"=w430, "estadoTorre"=w469) -> ("¿disponible?"=w425:bool, "posicionCero"=w468:i32)
        n291 = call "estadoTorre.vi"("¿pieza?"=w431, "estadoTorre"=w472) -> ("¿disponible?"=w427:bool, "posicionCero"=w471:i32)
        n292 = call "estadoTorre.vi"("¿pieza?"=w429, "estadoTorre"=w466) -> ("¿disponible?"=w423:bool, "posicionCero"=w465:i32)
        n293 = Bundle(w444, "Top"=w443) -> (w445:cluster{u32, "Top":i32})  [unwired: 1 in]
        n294 = Bundle("Left"=w440, w441) -> (w439:cluster{"Left":i32, u32})  [unwired: 1 in]
        n295 = Bundle(w455, "Top"=w453) -> (w454:cluster{u32, "Top":i32})  [unwired: 1 in]
        n296 = Bundle("Left"=w450, w451) -> (w449:cluster{"Left":i32, u32})  [unwired: 1 in]
        n297 = Bundle(w464, "Top"=w460) -> (w433:cluster{u32, "Top":i32})  [unwired: 1 in]
        n298 = Bundle("Left"=w458, w457) -> (w435:cluster{"Left":i32, u32})  [unwired: 1 in]
        n299 = call "perteneceAtorre.vi"("P1"=w438, "P2"=w445, "P"=w474, "P3"=w439, "P4"=w436) -> ("out"=w424:bool)
        n300 = call "perteneceAtorre.vi"("P1"=w447, "P2"=w454, "P"=w474, "P3"=w446, "P4"=w449) -> ("out"=w426:bool)
        n301 = call "perteneceAtorre.vi"("P1"=w462, "P2"=w433, "P"=w474, "P3"=w461, "P4"=w435) -> ("out"=w428:bool)
        n302 = And(x=w424, y=w423) -> (x .and. y?=w467:bool)
        n303 = And(x=w428, y=w427) -> (x .and. y?=w473:bool)
        n304 = And(x=w426, y=w425) -> (x .and. y?=w470:bool)
        n305 = case shown="False" w473 {
          tunnel: w471 -> [_ w652]
          tunnel: w472 -> [_ w651]
          tunnel: w470 -> [w482 _]
          tunnel: w468 -> [w481 _]
          tunnel: w469 -> [w480 _]
          tunnel: w467 -> [w479 _]
          tunnel: w465 -> [w478 _]
          tunnel: w466 -> [w477 _]
          frame False {
            n306 = case shown="False" w482 {
              tunnel: w481 -> [_ w573]
              tunnel: w480 -> [_ w572]
              tunnel: w479 -> [w485 _]
              tunnel: w478 -> [w484 _]
              tunnel: w477 -> [w483 _]
              frame False {
                n307 = case shown="False" w485 {
                  tunnel: w484 -> [_ w492]
                  tunnel: w483 -> [_ w493]
                  frame False {
                    n308 = local read "PosAntPiezaCuatro"() -> (w486:T1)
                    n309 = property on="PiezaCuatro" class="Bool (strict)"("Position"=w486) -> ()  [unwired: 2 in, 2 out]
                  }
                  frame True {
                    n310 = local read "Torre"() -> (w490:i8)
                    n311 = local read "numPiezas"() -> (w500:enum16{"5", "4", "3"})
                    n312 = Equal?(x=w490, y=i8 1) -> (x = y?=w491:bool)
                    n313 = case shown="False" w491 {
                      tunnel: w490 -> [w505 _]
                      frame False {
                        n314 = Equal?(x=w505, y=i8 2) -> (x = y?=w506:bool)
                        n315 = case shown="False" w506 {
                          frame False {
                            n316 = local read "estadoTorreTres"() -> (w511:i32[])
                            n317 = Search 1D Array(1D array=w511, element=0) -> (index of element=w510:i32)  [unwired: 1 in]
                            n318 = Equal?(x=w510, y=-1) -> (x = y?=w512:bool)
                            n319 = case shown="False" w512 {
                              tunnel: w511 -> [w513 w524]
                              tunnel: w510 -> [w514 _]
                              frame False {
                                n320 = Equal?(x=w514, y=0) -> (x = y?=w515:bool)
                                n321 = case shown="False" w515 {
                                tunnel: w514 -> [w521 _]
                                tunnel: w513 -> [w519 _]
                                frame False {
                                n322 = Decrement(x=w521) -> (x-1=w520:i32)
                                n323 = Replace Array Subset(array=w519, new element=0 ("new element/subarray"), index=w520) -> (w517:i32[])
                                n324 = local write "estadoTorreTres"(w517) -> ()
                                }
                                frame True {
                                }
                                }
                              }
                              frame True {
                                n325 = Array Size(array=w524) -> (size(s)=w526:i32)
                                n326 = Decrement(x=w526) -> (x-1=w525:i32)
                                n327 = Replace Array Subset(array=w524, new element=0 ("new element/subarray"), index=w525) -> (w522:i32[])
                                n328 = local write "estadoTorreTres"(w522) -> ()
                              }
                            }
                          }
                          frame True {
                            n329 = local read "estadoTorreDos"() -> (w528:i32[])
                            n330 = Search 1D Array(1D array=w528, element=0) -> (index of element=w527:i32)  [unwired: 1 in]
                            n331 = Equal?(x=w527, y=-1) -> (x = y?=w529:bool)
                            n332 = case shown="True" w529 {
                              tunnel: w528 -> [w532 w543]
                              tunnel: w527 -> [w533 _]
                              frame False {
                                n333 = Equal?(x=w533, y=0) -> (x = y?=w534:bool)
                                n334 = case shown="True" w534 {
                                tunnel: w533 -> [w540 _]
                                tunnel: w532 -> [w538 _]
                                frame False {
                                n335 = Decrement(x=w540) -> (x-1=w539:i32)
                                n336 = Replace Array Subset(array=w538, new element=0 ("new element/subarray"), index=w539) -> (w536:i32[])
                                n337 = local write "estadoTorreDos"(w536) -> ()
                                }
                                frame True {
                                }
                                }
                              }
                              frame True {
                                n338 = Array Size(array=w543) -> (size(s)=w545:i32)
                                n339 = Decrement(x=w545) -> (x-1=w544:i32)
                                n340 = Replace Array Subset(array=w543, new element=0 ("new element/subarray"), index=w544) -> (w541:i32[])
                                n341 = local write "estadoTorreDos"(w541) -> ()
                              }
                            }
                          }
                        }
                      }
                      frame True {
                        n342 = local read "estadoTorreUno"() -> (w547:i32[])
                        n343 = Search 1D Array(1D array=w547, element=0) -> (index of element=w546:i32)  [unwired: 1 in]
                        n344 = Equal?(x=w546, y=-1) -> (x = y?=w548:bool)
                        n345 = case shown="False" w548 {
                          tunnel: w547 -> [w551 w562]
                          tunnel: w546 -> [w552 _]
                          frame False {
                            n346 = Equal?(x=w552, y=0) -> (x = y?=w553:bool)
                            n347 = case shown="False" w553 {
                              tunnel: w552 -> [w559 _]
                              tunnel: w551 -> [w557 _]
                              frame False {
                                n348 = Decrement(x=w559) -> (x-1=w558:i32)
                                n349 = Replace Array Subset(array=w557, new element=0 ("new element/subarray"), index=w558) -> (w555:i32[])
                                n350 = local write "estadoTorreUno"(w555) -> ()
                              }
                              frame True {
                              }
                            }
                          }
                          frame True {
                            n351 = Array Size(array=w562) -> (size(s)=w564:i32)
                            n352 = Decrement(x=w564) -> (x-1=w563:i32)
                            n353 = Replace Array Subset(array=w562, new element=0 ("new element/subarray"), index=w563) -> (w560:i32[])
                            n354 = local write "estadoTorreUno"(w560) -> ()
                          }
                        }
                      }
                    }
                    n355 = call "auxiliar.vi"("posicion"=w492, "numPiezas"=w500) -> ("posicion"=w499:i32)
                    n356 = Replace Array Subset(array=w493, new element=4, index=w492) -> (w504:i32[])
                    n357 = Decrement(x=w499) -> (x-1=w488:i32)
                    n358 = local read "posPiezaCuatro"() -> (w503:i32[][])
                    n359 = local write "estadoTorreUno"(w504) -> ()
                    n360 = Index Array(array=w503, index (row) #1=w488, index (col) #1=0 ("disabled index (col)"), index (row) #2=w488, index (col) #2=1 ("disabled index (col)")) -> (element #1=w502:i32, element #2=w501:i32)
                    n361 = local read "numMov"() -> (w498:dbl)
                    n362 = Bundle(w502, w501) -> (w487:cluster{i32, i32})  [unwired: 1 in]
                    n363 = Increment(x=w498) -> (x+1=w497:dbl)
                    n364 = property on="PiezaCuatro" class="Bool (strict)"("Position"=w487) -> ()  [unwired: 2 in, 2 out]
                    n365 = local write "numMov"(w497) -> ()
                  }
                }
              }
              frame True {
                n366 = local read "numPiezas"() -> (w579:enum16{"5", "4", "3"})
                n367 = local read "Torre"() -> (w569:i8)
                n368 = Equal?(x=w569, y=i8 1) -> (x = y?=w571:bool)
                n369 = call "auxiliar.vi"("posicion"=w573, "numPiezas"=w579) -> ("posicion"=w567:i32)
                n370 = case shown="False" w571 {
                  tunnel: w569 -> [w584 _]
                  frame False {
                    n371 = Equal?(x=w584, y=i8 2) -> (x = y?=w585:bool)
                    n372 = case shown="True" w585 {
                      frame False {
                        n373 = local read "estadoTorreTres"() -> (w590:i32[])
                        n374 = Search 1D Array(1D array=w590, element=0) -> (index of element=w589:i32)  [unwired: 1 in]
                        n375 = Equal?(x=w589, y=-1) -> (x = y?=w591:bool)
                        n376 = case shown="False" w591 {
                          tunnel: w590 -> [w592 w603]
                          tunnel: w589 -> [w593 _]
                          frame False {
                            n377 = Equal?(x=w593, y=0) -> (x = y?=w594:bool)
                            n378 = case shown="True" w594 {
                              tunnel: w593 -> [w600 _]
                              tunnel: w592 -> [w598 _]
                              frame False {
                                n379 = Decrement(x=w600) -> (x-1=w599:i32)
                                n380 = Replace Array Subset(array=w598, new element=0 ("new element/subarray"), index=w599) -> (w596:i32[])
                                n381 = local write "estadoTorreTres"(w596) -> ()
                              }
                              frame True {
                              }
                            }
                          }
                          frame True {
                            n382 = Array Size(array=w603) -> (size(s)=w605:i32)
                            n383 = Decrement(x=w605) -> (x-1=w604:i32)
                            n384 = Replace Array Subset(array=w603, new element=0 ("new element/subarray"), index=w604) -> (w601:i32[])
                            n385 = local write "estadoTorreTres"(w601) -> ()
                          }
                        }
                      }
                      frame True {
                        n386 = local read "estadoTorreDos"() -> (w607:i32[])
                        n387 = Search 1D Array(1D array=w607, element=0) -> (index of element=w606:i32)  [unwired: 1 in]
                        n388 = Equal?(x=w606, y=-1) -> (x = y?=w608:bool)
                        n389 = case shown="True" w608 {
                          tunnel: w607 -> [w611 w622]
                          tunnel: w606 -> [w612 _]
                          frame False {
                            n390 = Equal?(x=w612, y=0) -> (x = y?=w613:bool)
                            n391 = case shown="True" w613 {
                              tunnel: w612 -> [w619 _]
                              tunnel: w611 -> [w617 _]
                              frame False {
                                n392 = Decrement(x=w619) -> (x-1=w618:i32)
                                n393 = Replace Array Subset(array=w617, new element=0 ("new element/subarray"), index=w618) -> (w615:i32[])
                                n394 = local write "estadoTorreDos"(w615) -> ()
                              }
                              frame True {
                              }
                            }
                          }
                          frame True {
                            n395 = Array Size(array=w622) -> (size(s)=w624:i32)
                            n396 = Decrement(x=w624) -> (x-1=w623:i32)
                            n397 = Replace Array Subset(array=w622, new element=0 ("new element/subarray"), index=w623) -> (w620:i32[])
                            n398 = local write "estadoTorreDos"(w620) -> ()
                          }
                        }
                      }
                    }
                  }
                  frame True {
                    n399 = local read "estadoTorreUno"() -> (w626:i32[])
                    n400 = Search 1D Array(1D array=w626, element=0) -> (index of element=w625:i32)  [unwired: 1 in]
                    n401 = Equal?(x=w625, y=-1) -> (x = y?=w627:bool)
                    n402 = case shown="False" w627 {
                      tunnel: w626 -> [w630 w641]
                      tunnel: w625 -> [w631 _]
                      frame False {
                        n403 = Equal?(x=w631, y=0) -> (x = y?=w632:bool)
                        n404 = case shown="False" w632 {
                          tunnel: w631 -> [w638 _]
                          tunnel: w630 -> [w636 _]
                          frame False {
                            n405 = Decrement(x=w638) -> (x-1=w637:i32)
                            n406 = Replace Array Subset(array=w636, new element=0 ("new element/subarray"), index=w637) -> (w634:i32[])
                            n407 = local write "estadoTorreUno"(w634) -> ()
                          }
                          frame True {
                          }
                        }
                      }
                      frame True {
                        n408 = Array Size(array=w641) -> (size(s)=w643:i32)
                        n409 = Decrement(x=w643) -> (x-1=w642:i32)
                        n410 = Replace Array Subset(array=w641, new element=0 ("new element/subarray"), index=w642) -> (w639:i32[])
                        n411 = local write "estadoTorreUno"(w639) -> ()
                      }
                    }
                  }
                }
                n412 = Replace Array Subset(array=w572, new element=4, index=w573) -> (w583:i32[])
                n413 = Subtract(x=w567, y=3) -> (x-y=w568:i32)
                n414 = local read "posPiezaCuatro"() -> (w582:i32[][])
                n415 = local write "estadoTorreTres"(w583) -> ()
                n416 = Index Array(array=w582, index (row) #1=w568, index (col) #1=4 ("disabled index (col)"), index (row) #2=w568, index (col) #2=5 ("disabled index (col)")) -> (element #1=w581:i32, element #2=w580:i32)
                n417 = local read "numMov"() -> (w578:dbl)
                n418 = Bundle(w581, w580) -> (w565:cluster{i32, i32})  [unwired: 1 in]
                n419 = Increment(x=w578) -> (x+1=w577:dbl)
                n420 = property on="PiezaCuatro" class="Bool (strict)"("Position"=w565) -> ()  [unwired: 2 in, 2 out]
                n421 = local write "numMov"(w577) -> ()
              }
            }
          }
          frame True {
            n422 = local read "numPiezas"() -> (w658:enum16{"5", "4", "3"})
            n423 = local read "Torre"() -> (w648:i8)
            n424 = Equal?(x=w648, y=i8 1) -> (x = y?=w650:bool)
            n425 = call "auxiliar.vi"("posicion"=w652, "numPiezas"=w658) -> ("posicion"=w646:i32)
            n426 = case shown="False" w650 {
              tunnel: w648 -> [w663 _]
              frame False {
                n427 = Equal?(x=w663, y=i8 2) -> (x = y?=w664:bool)
                n428 = case shown="False" w664 {
                  frame False {
                    n429 = local read "estadoTorreTres"() -> (w669:i32[])
                    n430 = Search 1D Array(1D array=w669, element=0) -> (index of element=w668:i32)  [unwired: 1 in]
                    n431 = Equal?(x=w668, y=-1) -> (x = y?=w670:bool)
                    n432 = case shown="False" w670 {
                      tunnel: w669 -> [w671 w682]
                      tunnel: w668 -> [w672 _]
                      frame False {
                        n433 = Equal?(x=w672, y=0) -> (x = y?=w673:bool)
                        n434 = case shown="False" w673 {
                          tunnel: w672 -> [w679 _]
                          tunnel: w671 -> [w677 _]
                          frame False {
                            n435 = Decrement(x=w679) -> (x-1=w678:i32)
                            n436 = Replace Array Subset(array=w677, new element=0 ("new element/subarray"), index=w678) -> (w675:i32[])
                            n437 = local write "estadoTorreTres"(w675) -> ()
                          }
                          frame True {
                          }
                        }
                      }
                      frame True {
                        n438 = Array Size(array=w682) -> (size(s)=w684:i32)
                        n439 = Decrement(x=w684) -> (x-1=w683:i32)
                        n440 = Replace Array Subset(array=w682, new element=0 ("new element/subarray"), index=w683) -> (w680:i32[])
                        n441 = local write "estadoTorreTres"(w680) -> ()
                      }
                    }
                  }
                  frame True {
                    n442 = local read "estadoTorreDos"() -> (w686:i32[])
                    n443 = Search 1D Array(1D array=w686, element=0) -> (index of element=w685:i32)  [unwired: 1 in]
                    n444 = Equal?(x=w685, y=-1) -> (x = y?=w687:bool)
                    n445 = case shown="True" w687 {
                      tunnel: w686 -> [w690 w701]
                      tunnel: w685 -> [w691 _]
                      frame False {
                        n446 = Equal?(x=w691, y=0) -> (x = y?=w692:bool)
                        n447 = case shown="True" w692 {
                          tunnel: w691 -> [w698 _]
                          tunnel: w690 -> [w696 _]
                          frame False {
                            n448 = Decrement(x=w698) -> (x-1=w697:i32)
                            n449 = Replace Array Subset(array=w696, new element=0 ("new element/subarray"), index=w697) -> (w694:i32[])
                            n450 = local write "estadoTorreDos"(w694) -> ()
                          }
                          frame True {
                          }
                        }
                      }
                      frame True {
                        n451 = Array Size(array=w701) -> (size(s)=w703:i32)
                        n452 = Decrement(x=w703) -> (x-1=w702:i32)
                        n453 = Replace Array Subset(array=w701, new element=0 ("new element/subarray"), index=w702) -> (w699:i32[])
                        n454 = local write "estadoTorreDos"(w699) -> ()
                      }
                    }
                  }
                }
              }
              frame True {
                n455 = local read "estadoTorreUno"() -> (w705:i32[])
                n456 = Search 1D Array(1D array=w705, element=0) -> (index of element=w704:i32)  [unwired: 1 in]
                n457 = Equal?(x=w704, y=-1) -> (x = y?=w706:bool)
                n458 = case shown="False" w706 {
                  tunnel: w705 -> [w709 w720]
                  tunnel: w704 -> [w710 _]
                  frame False {
                    n459 = Equal?(x=w710, y=0) -> (x = y?=w711:bool)
                    n460 = case shown="False" w711 {
                      tunnel: w710 -> [w717 _]
                      tunnel: w709 -> [w715 _]
                      frame False {
                        n461 = Decrement(x=w717) -> (x-1=w716:i32)
                        n462 = Replace Array Subset(array=w715, new element=0 ("new element/subarray"), index=w716) -> (w713:i32[])
                        n463 = local write "estadoTorreUno"(w713) -> ()
                      }
                      frame True {
                      }
                    }
                  }
                  frame True {
                    n464 = Array Size(array=w720) -> (size(s)=w722:i32)
                    n465 = Decrement(x=w722) -> (x-1=w721:i32)
                    n466 = Replace Array Subset(array=w720, new element=0 ("new element/subarray"), index=w721) -> (w718:i32[])
                    n467 = local write "estadoTorreUno"(w718) -> ()
                  }
                }
              }
            }
            n468 = Replace Array Subset(array=w651, new element=4, index=w652) -> (w662:i32[])
            n469 = Subtract(x=w646, y=3) -> (x-y=w647:i32)
            n470 = local read "posPiezaCuatro"() -> (w661:i32[][])
            n471 = local write "estadoTorreDos"(w662) -> ()
            n472 = Index Array(array=w661, index (row) #1=w647, index (col) #1=2 ("disabled index (col)"), index (row) #2=w647, index (col) #2=3 ("disabled index (col)")) -> (element #1=w660:i32, element #2=w659:i32)
            n473 = local read "numMov"() -> (w657:dbl)
            n474 = Bundle(w660, w659) -> (w644:cluster{i32, i32})  [unwired: 1 in]
            n475 = Increment(x=w657) -> (x+1=w656:dbl)
            n476 = property on="PiezaCuatro" class="Bool (strict)"("Position"=w644) -> ()  [unwired: 2 in, 2 out]
            n477 = local write "numMov"(w656) -> ()
          }
        }
      }
      event "Deterner": Value Change {
        n478 = event-data() -> ()  [unwired: 1 in, 6 out]
      }
      event "PiezaCinco": Mouse Up {
        n479 = event-data() -> ("Coords"=w775:T4)  [unwired: 1 in]
        n480 = property on="TorreUno" class="Slide (strict)"() -> ("Position"=w739:T1, "Left"=w741:i32, "Top"=w744:i32, "Bounds"=w738:T3, "Height"=w743:u32, "Width"=w733:u32)  [unwired: 2 in, 2 out]
        n481 = property on="TorreTres" class="Slide (strict)"() -> ("Position"=w748:T1, "Left"=w751:i32, "Top"=w754:i32, "Bounds"=w749:T3, "Height"=w753:u32, "Width"=w757:u32)  [unwired: 2 in, 2 out]
        n482 = property on="TorreDos" class="Slide (strict)"() -> ("Position"=w763:T1, "Left"=w759:i32, "Top"=w761:i32, "Bounds"=w764:T3, "Height"=w760:u32, "Width"=w735:u32)  [unwired: 2 in, 2 out]
        n483 = local read "estadoTorreTres"() -> (w770:i32[])
        n484 = local read "estadoTorreDos"() -> (w773:i32[])
        n485 = local read "estadoTorreUno"() -> (w767:i32[])
        n486 = local read "¿Pieza?"() -> (w731:i8)
        n487 = local read "¿Pieza?"() -> (w732:i8)
        n488 = local read "¿Pieza?"() -> (w730:i8)
        n489 = Add(x=w741, y=w733) -> (x+y=w745:u32)
        n490 = Add(x=w744, y=w743) -> (x+y=w742:u32)
        n491 = Add(x=w739, y=w738) -> (x+y=w737:T3)
        n492 = Add(x=w751, y=w757) -> (x+y=w756:u32)
        n493 = Add(x=w748, y=w749) -> (x+y=w747:T3)
        n494 = Add(x=w754, y=w753) -> (x+y=w752:u32)
        n495 = Add(x=w759, y=w735) -> (x+y=w765:u32)
        n496 = Add(x=w763, y=w764) -> (x+y=w762:T3)
        n497 = Add(x=w761, y=w760) -> (x+y=w758:u32)
        n498 = call "estadoTorre.vi"("¿pieza?"=w731, "estadoTorre"=w770) -> ("¿disponible?"=w726:bool, "posicionCero"=w769:i32)
        n499 = call "estadoTorre.vi"("¿pieza?"=w732, "estadoTorre"=w773) -> ("¿disponible?"=w728:bool, "posicionCero"=w772:i32)
        n500 = call "estadoTorre.vi"("¿pieza?"=w730, "estadoTorre"=w767) -> ("¿disponible?"=w724:bool, "posicionCero"=w766:i32)
        n501 = Bundle(w745, "Top"=w744) -> (w746:cluster{u32, "Top":i32})  [unwired: 1 in]
        n502 = Bundle("Left"=w741, w742) -> (w740:cluster{"Left":i32, u32})  [unwired: 1 in]
        n503 = Bundle(w756, "Top"=w754) -> (w755:cluster{u32, "Top":i32})  [unwired: 1 in]
        n504 = Bundle("Left"=w751, w752) -> (w750:cluster{"Left":i32, u32})  [unwired: 1 in]
        n505 = Bundle(w765, "Top"=w761) -> (w734:cluster{u32, "Top":i32})  [unwired: 1 in]
        n506 = Bundle("Left"=w759, w758) -> (w736:cluster{"Left":i32, u32})  [unwired: 1 in]
        n507 = call "perteneceAtorre.vi"("P1"=w739, "P2"=w746, "P"=w775, "P3"=w740, "P4"=w737) -> ("out"=w725:bool)
        n508 = call "perteneceAtorre.vi"("P1"=w748, "P2"=w755, "P"=w775, "P3"=w747, "P4"=w750) -> ("out"=w727:bool)
        n509 = call "perteneceAtorre.vi"("P1"=w763, "P2"=w734, "P"=w775, "P3"=w762, "P4"=w736) -> ("out"=w729:bool)
        n510 = And(x=w725, y=w724) -> (x .and. y?=w768:bool)
        n511 = And(x=w729, y=w728) -> (x .and. y?=w774:bool)
        n512 = And(x=w727, y=w726) -> (x .and. y?=w771:bool)
        n513 = case shown="False" w774 {
          tunnel: w772 -> [_ w943]
          tunnel: w773 -> [_ w942]
          tunnel: w771 -> [w781 _]
          tunnel: w769 -> [w780 _]
          tunnel: w770 -> [w779 _]
          tunnel: w768 -> [w778 _]
          tunnel: w766 -> [w777 _]
          tunnel: w767 -> [w776 _]
          frame False {
            n514 = case shown="False" w781 {
              tunnel: w780 -> [_ w868]
              tunnel: w779 -> [_ w867]
              tunnel: w778 -> [w784 _]
              tunnel: w777 -> [w783 _]
              tunnel: w776 -> [w782 _]
              frame False {
                n515 = case shown="True" w784 {
                  tunnel: w783 -> [_ w792]
                  tunnel: w782 -> [_ w793]
                  frame False {
                    n516 = local read "PosAntPiezaCinco"() -> (w785:T1)
                    n517 = property on="PiezaCinco" class="Bool (strict)"("Position"=w785) -> ()  [unwired: 2 in, 2 out]
                  }
                  frame True {
                    n518 = local read "Torre"() -> (w790:i8)
                    n519 = Equal?(x=w790, y=i8 1) -> (x = y?=w791:bool)
                    n520 = case shown="False" w791 {
                      tunnel: w790 -> [w801 _]
                      frame False {
                        n521 = Equal?(x=w801, y=i8 2) -> (x = y?=w802:bool)
                        n522 = case shown="False" w802 {
                          frame False {
                            n523 = local read "estadoTorreTres"() -> (w807:i32[])
                            n524 = Search 1D Array(1D array=w807, element=0) -> (index of element=w806:i32)  [unwired: 1 in]
                            n525 = Equal?(x=w806, y=-1) -> (x = y?=w808:bool)
                            n526 = case shown="False" w808 {
                              tunnel: w807 -> [w809 w820]
                              tunnel: w806 -> [w810 _]
                              frame False {
                                n527 = Equal?(x=w810, y=0) -> (x = y?=w811:bool)
                                n528 = case shown="False" w811 {
                                tunnel: w810 -> [w817 _]
                                tunnel: w809 -> [w815 _]
                                frame False {
                                n529 = Decrement(x=w817) -> (x-1=w816:i32)
                                n530 = Replace Array Subset(array=w815, new element=0 ("new element/subarray"), index=w816) -> (w813:i32[])
                                n531 = local write "estadoTorreTres"(w813) -> ()
                                }
                                frame True {
                                }
                                }
                              }
                              frame True {
                                n532 = Array Size(array=w820) -> (size(s)=w822:i32)
                                n533 = Decrement(x=w822) -> (x-1=w821:i32)
                                n534 = Replace Array Subset(array=w820, new element=0 ("new element/subarray"), index=w821) -> (w818:i32[])
                                n535 = local write "estadoTorreTres"(w818) -> ()
                              }
                            }
                          }
                          frame True {
                            n536 = local read "estadoTorreDos"() -> (w824:i32[])
                            n537 = Search 1D Array(1D array=w824, element=0) -> (index of element=w823:i32)  [unwired: 1 in]
                            n538 = Equal?(x=w823, y=-1) -> (x = y?=w825:bool)
                            n539 = case shown="True" w825 {
                              tunnel: w824 -> [w828 w839]
                              tunnel: w823 -> [w829 _]
                              frame False {
                                n540 = Equal?(x=w829, y=0) -> (x = y?=w830:bool)
                                n541 = case shown="True" w830 {
                                tunnel: w829 -> [w836 _]
                                tunnel: w828 -> [w834 _]
                                frame False {
                                n542 = Decrement(x=w836) -> (x-1=w835:i32)
                                n543 = Replace Array Subset(array=w834, new element=0 ("new element/subarray"), index=w835) -> (w832:i32[])
                                n544 = local write "estadoTorreDos"(w832) -> ()
                                }
                                frame True {
                                }
                                }
                              }
                              frame True {
                                n545 = Array Size(array=w839) -> (size(s)=w841:i32)
                                n546 = Decrement(x=w841) -> (x-1=w840:i32)
                                n547 = Replace Array Subset(array=w839, new element=0 ("new element/subarray"), index=w840) -> (w837:i32[])
                                n548 = local write "estadoTorreDos"(w837) -> ()
                              }
                            }
                          }
                        }
                      }
                      frame True {
                        n549 = local read "estadoTorreUno"() -> (w843:i32[])
                        n550 = Search 1D Array(1D array=w843, element=0) -> (index of element=w842:i32)  [unwired: 1 in]
                        n551 = Equal?(x=w842, y=-1) -> (x = y?=w844:bool)
                        n552 = case shown="False" w844 {
                          tunnel: w843 -> [w847 w858]
                          tunnel: w842 -> [w848 _]
                          frame False {
                            n553 = Equal?(x=w848, y=0) -> (x = y?=w849:bool)
                            n554 = case shown="False" w849 {
                              tunnel: w848 -> [w855 _]
                              tunnel: w847 -> [w853 _]
                              frame False {
                                n555 = Decrement(x=w855) -> (x-1=w854:i32)
                                n556 = Replace Array Subset(array=w853, new element=0 ("new element/subarray"), index=w854) -> (w851:i32[])
                                n557 = local write "estadoTorreUno"(w851) -> ()
                              }
                              frame True {
                              }
                            }
                          }
                          frame True {
                            n558 = Array Size(array=w858) -> (size(s)=w860:i32)
                            n559 = Decrement(x=w860) -> (x-1=w859:i32)
                            n560 = Replace Array Subset(array=w858, new element=0 ("new element/subarray"), index=w859) -> (w856:i32[])
                            n561 = local write "estadoTorreUno"(w856) -> ()
                          }
                        }
                      }
                    }
                    n562 = Replace Array Subset(array=w793, new element=5, index=w792) -> (w800:i32[])
                    n563 = local write "estadoTorreUno"(w800) -> ()
                    n564 = local read "posPiezaCinco"() -> (w799:i32[])
                    n565 = Index Array(array=w799, index #1=0 ("index"), index #2=1 ("index")) -> (element #1=w798:i32, element #2=w797:i32)
                    n566 = local read "numMov"() -> (w796:dbl)
                    n567 = Bundle(w798, w797) -> (w786:cluster{i32, i32})  [unwired: 1 in]
                    n568 = Increment(x=w796) -> (x+1=w795:dbl)
                    n569 = property on="PiezaCinco" class="Bool (strict)"("Position"=w786) -> ()  [unwired: 2 in, 2 out]
                    n570 = local write "numMov"(w795) -> ()
                  }
                }
              }
              frame True {
                n571 = local read "Torre"() -> (w864:i8)
                n572 = Equal?(x=w864, y=i8 1) -> (x = y?=w866:bool)
                n573 = case shown="False" w866 {
                  tunnel: w864 -> [w876 _]
                  frame False {
                    n574 = Equal?(x=w876, y=i8 2) -> (x = y?=w877:bool)
                    n575 = case shown="True" w877 {
                      frame False {
                        n576 = local read "estadoTorreTres"() -> (w882:i32[])
                        n577 = Search 1D Array(1D array=w882, element=0) -> (index of element=w881:i32)  [unwired: 1 in]
                        n578 = Equal?(x=w881, y=-1) -> (x = y?=w883:bool)
                        n579 = case shown="False" w883 {
                          tunnel: w882 -> [w884 w895]
                          tunnel: w881 -> [w885 _]
                          frame False {
                            n580 = Equal?(x=w885, y=0) -> (x = y?=w886:bool)
                            n581 = case shown="True" w886 {
                              tunnel: w885 -> [w892 _]
                              tunnel: w884 -> [w890 _]
                              frame False {
                                n582 = Decrement(x=w892) -> (x-1=w891:i32)
                                n583 = Replace Array Subset(array=w890, new element=0 ("new element/subarray"), index=w891) -> (w888:i32[])
                                n584 = local write "estadoTorreTres"(w888) -> ()
                              }
                              frame True {
                              }
                            }
                          }
                          frame True {
                            n585 = Array Size(array=w895) -> (size(s)=w897:i32)
                            n586 = Decrement(x=w897) -> (x-1=w896:i32)
                            n587 = Replace Array Subset(array=w895, new element=0 ("new element/subarray"), index=w896) -> (w893:i32[])
                            n588 = local write "estadoTorreTres"(w893) -> ()
                          }
                        }
                      }
                      frame True {
                        n589 = local read "estadoTorreDos"() -> (w899:i32[])
                        n590 = Search 1D Array(1D array=w899, element=0) -> (index of element=w898:i32)  [unwired: 1 in]
                        n591 = Equal?(x=w898, y=-1) -> (x = y?=w900:bool)
                        n592 = case shown="True" w900 {
                          tunnel: w899 -> [w903 w914]
                          tunnel: w898 -> [w904 _]
                          frame False {
                            n593 = Equal?(x=w904, y=0) -> (x = y?=w905:bool)
                            n594 = case shown="True" w905 {
                              tunnel: w904 -> [w911 _]
                              tunnel: w903 -> [w909 _]
                              frame False {
                                n595 = Decrement(x=w911) -> (x-1=w910:i32)
                                n596 = Replace Array Subset(array=w909, new element=0 ("new element/subarray"), index=w910) -> (w907:i32[])
                                n597 = local write "estadoTorreDos"(w907) -> ()
                              }
                              frame True {
                              }
                            }
                          }
                          frame True {
                            n598 = Array Size(array=w914) -> (size(s)=w916:i32)
                            n599 = Decrement(x=w916) -> (x-1=w915:i32)
                            n600 = Replace Array Subset(array=w914, new element=0 ("new element/subarray"), index=w915) -> (w912:i32[])
                            n601 = local write "estadoTorreDos"(w912) -> ()
                          }
                        }
                      }
                    }
                  }
                  frame True {
                    n602 = local read "estadoTorreUno"() -> (w918:i32[])
                    n603 = Search 1D Array(1D array=w918, element=0) -> (index of element=w917:i32)  [unwired: 1 in]
                    n604 = Equal?(x=w917, y=-1) -> (x = y?=w919:bool)
                    n605 = case shown="False" w919 {
                      tunnel: w918 -> [w922 w933]
                      tunnel: w917 -> [w923 _]
                      frame False {
                        n606 = Equal?(x=w923, y=0) -> (x = y?=w924:bool)
                        n607 = case shown="False" w924 {
                          tunnel: w923 -> [w930 _]
                          tunnel: w922 -> [w928 _]
                          frame False {
                            n608 = Decrement(x=w930) -> (x-1=w929:i32)
                            n609 = Replace Array Subset(array=w928, new element=0 ("new element/subarray"), index=w929) -> (w926:i32[])
                            n610 = local write "estadoTorreUno"(w926) -> ()
                          }
                          frame True {
                          }
                        }
                      }
                      frame True {
                        n611 = Array Size(array=w933) -> (size(s)=w935:i32)
                        n612 = Decrement(x=w935) -> (x-1=w934:i32)
                        n613 = Replace Array Subset(array=w933, new element=0 ("new element/subarray"), index=w934) -> (w931:i32[])
                        n614 = local write "estadoTorreUno"(w931) -> ()
                      }
                    }
                  }
                }
                n615 = Replace Array Subset(array=w867, new element=5, index=w868) -> (w875:i32[])
                n616 = local read "posPiezaCinco"() -> (w874:i32[])
                n617 = local write "estadoTorreTres"(w875) -> ()
                n618 = Index Array(array=w874, index #1=4 ("disabled index (col)"), index #2=5 ("disabled index (col)")) -> (element #1=w873:i32, element #2=w872:i32)
                n619 = local read "numMov"() -> (w871:dbl)
                n620 = Bundle(w873, w872) -> (w863:cluster{i32, i32})  [unwired: 1 in]
                n621 = property on="PiezaCinco" class="Bool (strict)"("Position"=w863) -> ()  [unwired: 2 in, 2 out]
                n622 = Increment(x=w871) -> (x+1=w870:dbl)
                n623 = local write "numMov"(w870) -> ()
              }
            }
          }
          frame True {
            n624 = local read "Torre"() -> (w939:i8)
            n625 = Equal?(x=w939, y=i8 1) -> (x = y?=w941:bool)
            n626 = case shown="False" w941 {
              tunnel: w939 -> [w951 _]
              frame False {
                n627 = Equal?(x=w951, y=i8 2) -> (x = y?=w952:bool)
                n628 = case shown="False" w952 {
                  frame False {
                    n629 = local read "estadoTorreTres"() -> (w957:i32[])
                    n630 = Search 1D Array(1D array=w957, element=0) -> (index of element=w956:i32)  [unwired: 1 in]
                    n631 = Equal?(x=w956, y=-1) -> (x = y?=w958:bool)
                    n632 = case shown="False" w958 {
                      tunnel: w957 -> [w959 w970]
                      tunnel: w956 -> [w960 _]
                      frame False {
                        n633 = Equal?(x=w960, y=0) -> (x = y?=w961:bool)
                        n634 = case shown="False" w961 {
                          tunnel: w960 -> [w967 _]
                          tunnel: w959 -> [w965 _]
                          frame False {
                            n635 = Decrement(x=w967) -> (x-1=w966:i32)
                            n636 = Replace Array Subset(array=w965, new element=0 ("new element/subarray"), index=w966) -> (w963:i32[])
                            n637 = local write "estadoTorreTres"(w963) -> ()
                          }
                          frame True {
                          }
                        }
                      }
                      frame True {
                        n638 = Array Size(array=w970) -> (size(s)=w972:i32)
                        n639 = Decrement(x=w972) -> (x-1=w971:i32)
                        n640 = Replace Array Subset(array=w970, new element=0 ("new element/subarray"), index=w971) -> (w968:i32[])
                        n641 = local write "estadoTorreTres"(w968) -> ()
                      }
                    }
                  }
                  frame True {
                    n642 = local read "estadoTorreDos"() -> (w974:i32[])
                    n643 = Search 1D Array(1D array=w974, element=0) -> (index of element=w973:i32)  [unwired: 1 in]
                    n644 = Equal?(x=w973, y=-1) -> (x = y?=w975:bool)
                    n645 = case shown="True" w975 {
                      tunnel: w974 -> [w978 w989]
                      tunnel: w973 -> [w979 _]
                      frame False {
                        n646 = Equal?(x=w979, y=0) -> (x = y?=w980:bool)
                        n647 = case shown="True" w980 {
                          tunnel: w979 -> [w986 _]
                          tunnel: w978 -> [w984 _]
                          frame False {
                            n648 = Decrement(x=w986) -> (x-1=w985:i32)
                            n649 = Replace Array Subset(array=w984, new element=0 ("new element/subarray"), index=w985) -> (w982:i32[])
                            n650 = local write "estadoTorreDos"(w982) -> ()
                          }
                          frame True {
                          }
                        }
                      }
                      frame True {
                        n651 = Array Size(array=w989) -> (size(s)=w991:i32)
                        n652 = Decrement(x=w991) -> (x-1=w990:i32)
                        n653 = Replace Array Subset(array=w989, new element=0 ("new element/subarray"), index=w990) -> (w987:i32[])
                        n654 = local write "estadoTorreDos"(w987) -> ()
                      }
                    }
                  }
                }
              }
              frame True {
                n655 = local read "estadoTorreUno"() -> (w993:i32[])
                n656 = Search 1D Array(1D array=w993, element=0) -> (index of element=w992:i32)  [unwired: 1 in]
                n657 = Equal?(x=w992, y=-1) -> (x = y?=w994:bool)
                n658 = case shown="False" w994 {
                  tunnel: w993 -> [w997 w1008]
                  tunnel: w992 -> [w998 _]
                  frame False {
                    n659 = Equal?(x=w998, y=0) -> (x = y?=w999:bool)
                    n660 = case shown="False" w999 {
                      tunnel: w998 -> [w1005 _]
                      tunnel: w997 -> [w1003 _]
                      frame False {
                        n661 = Decrement(x=w1005) -> (x-1=w1004:i32)
                        n662 = Replace Array Subset(array=w1003, new element=0 ("new element/subarray"), index=w1004) -> (w1001:i32[])
                        n663 = local write "estadoTorreUno"(w1001) -> ()
                      }
                      frame True {
                      }
                    }
                  }
                  frame True {
                    n664 = Array Size(array=w1008) -> (size(s)=w1010:i32)
                    n665 = Decrement(x=w1010) -> (x-1=w1009:i32)
                    n666 = Replace Array Subset(array=w1008, new element=0 ("new element/subarray"), index=w1009) -> (w1006:i32[])
                    n667 = local write "estadoTorreUno"(w1006) -> ()
                  }
                }
              }
            }
            n668 = Replace Array Subset(array=w942, new element=5, index=w943) -> (w950:i32[])
            n669 = local write "estadoTorreDos"(w950) -> ()
            n670 = local read "posPiezaCinco"() -> (w949:i32[])
            n671 = Index Array(array=w949, index #1=2 ("disabled index (col)"), index #2=3 ("disabled index (col)")) -> (element #1=w948:i32, element #2=w947:i32)
            n672 = local read "numMov"() -> (w946:dbl)
            n673 = Bundle(w948, w947) -> (w938:cluster{i32, i32})  [unwired: 1 in]
            n674 = Increment(x=w946) -> (x+1=w945:dbl)
            n675 = property on="PiezaCinco" class="Bool (strict)"("Position"=w938) -> ()  [unwired: 2 in, 2 out]
            n676 = local write "numMov"(w945) -> ()
          }
        }
      }
      event "PiezaDos": Mouse Up {
        n677 = event-data() -> ("Coords"=w1062:T4)  [unwired: 1 in]
        n678 = property on="TorreUno" class="Slide (strict)"() -> ("Position"=w1026:T1, "Left"=w1028:i32, "Top"=w1031:i32, "Bounds"=w1025:T3, "Height"=w1030:u32, "Width"=w1020:u32)  [unwired: 2 in, 2 out]
        n679 = property on="TorreTres" class="Slide (strict)"() -> ("Position"=w1035:T1, "Left"=w1038:i32, "Top"=w1041:i32, "Bounds"=w1036:T3, "Height"=w1040:u32, "Width"=w1044:u32)  [unwired: 2 in, 2 out]
        n680 = property on="TorreDos" class="Slide (strict)"() -> ("Position"=w1050:T1, "Left"=w1046:i32, "Top"=w1048:i32, "Bounds"=w1051:T3, "Height"=w1047:u32, "Width"=w1022:u32)  [unwired: 2 in, 2 out]
        n681 = local read "estadoTorreTres"() -> (w1056:i32[])
        n682 = local read "estadoTorreDos"() -> (w1059:i32[])
        n683 = local read "estadoTorreUno"() -> (w1053:i32[])
        n684 = local read "¿Pieza?"() -> (w1018:i8)
        n685 = local read "¿Pieza?"() -> (w1019:i8)
        n686 = local read "¿Pieza?"() -> (w1017:i8)
        n687 = Add(x=w1028, y=w1020) -> (x+y=w1032:u32)
        n688 = Add(x=w1031, y=w1030) -> (x+y=w1029:u32)
        n689 = Add(x=w1026, y=w1025) -> (x+y=w1024:T3)
        n690 = Add(x=w1038, y=w1044) -> (x+y=w1043:u32)
        n691 = Add(x=w1035, y=w1036) -> (x+y=w1034:T3)
        n692 = Add(x=w1041, y=w1040) -> (x+y=w1039:u32)
        n693 = Add(x=w1046, y=w1022) -> (x+y=w1052:u32)
        n694 = Add(x=w1050, y=w1051) -> (x+y=w1049:T3)
        n695 = Add(x=w1048, y=w1047) -> (x+y=w1045:u32)
        n696 = call "estadoTorre.vi"("¿pieza?"=w1018, "estadoTorre"=w1056) -> ("¿disponible?"=w1013:bool, "posicionCero"=w1057:i32)
        n697 = call "estadoTorre.vi"("¿pieza?"=w1019, "estadoTorre"=w1059) -> ("¿disponible?"=w1015:bool, "posicionCero"=w1060:i32)
        n698 = call "estadoTorre.vi"("¿pieza?"=w1017, "estadoTorre"=w1053) -> ("¿disponible?"=w1011:bool, "posicionCero"=w1054:i32)
        n699 = Bundle(w1032, "Top"=w1031) -> (w1033:cluster{u32, "Top":i32})  [unwired: 1 in]
        n700 = Bundle("Left"=w1028, w1029) -> (w1027:cluster{"Left":i32, u32})  [unwired: 1 in]
        n701 = Bundle(w1043, "Top"=w1041) -> (w1042:cluster{u32, "Top":i32})  [unwired: 1 in]
        n702 = Bundle("Left"=w1038, w1039) -> (w1037:cluster{"Left":i32, u32})  [unwired: 1 in]
        n703 = Bundle(w1052, "Top"=w1048) -> (w1021:cluster{u32, "Top":i32})  [unwired: 1 in]
        n704 = Bundle("Left"=w1046, w1045) -> (w1023:cluster{"Left":i32, u32})  [unwired: 1 in]
        n705 = call "perteneceAtorre.vi"("P1"=w1026, "P2"=w1033, "P"=w1062, "P3"=w1027, "P4"=w1024) -> ("out"=w1012:bool)
        n706 = call "perteneceAtorre.vi"("P1"=w1035, "P2"=w1042, "P"=w1062, "P3"=w1034, "P4"=w1037) -> ("out"=w1014:bool)
        n707 = call "perteneceAtorre.vi"("P1"=w1050, "P2"=w1021, "P"=w1062, "P3"=w1049, "P4"=w1023) -> ("out"=w1016:bool)
        n708 = And(x=w1012, y=w1011) -> (x .and. y?=w1055:bool)
        n709 = And(x=w1016, y=w1015) -> (x .and. y?=w1061:bool)
        n710 = And(x=w1014, y=w1013) -> (x .and. y?=w1058:bool)
        n711 = case shown="False" w1061 {
          tunnel: w1060 -> [_ w1237]
          tunnel: w1059 -> [_ w1236]
          tunnel: w1058 -> [w1070 _]
          tunnel: w1057 -> [w1069 _]
          tunnel: w1056 -> [w1068 _]
          tunnel: w1055 -> [w1067 _]
          tunnel: w1054 -> [w1066 _]
          tunnel: w1053 -> [w1065 _]
          frame False {
            n712 = case shown="True" w1070 {
              tunnel: w1069 -> [_ w1158]
              tunnel: w1068 -> [_ w1157]
              tunnel: w1067 -> [w1073 _]
              tunnel: w1066 -> [w1072 _]
              tunnel: w1065 -> [w1071 _]
              frame False {
                n713 = case shown="True" w1073 {
                  tunnel: w1072 -> [_ w1079]
                  tunnel: w1071 -> [_ w1080]
                  frame False {
                    n714 = local read "PosAntPiezaDos"() -> (w1074:T1)
                    n715 = property on="PiezaDos" class="Bool (strict)"("Position"=w1074) -> ()  [unwired: 2 in, 2 out]
                  }
                  frame True {
                    n716 = local read "Torre"() -> (w1077:i8)
                    n717 = local read "numPiezas"() -> (w1088:enum16{"5", "4", "3"})
                    n718 = Equal?(x=w1077, y=i8 1) -> (x = y?=w1078:bool)
                    n719 = case shown="False" w1078 {
                      tunnel: w1077 -> [w1093 _]
                      frame False {
                        n720 = Equal?(x=w1093, y=i8 2) -> (x = y?=w1094:bool)
                        n721 = case shown="False" w1094 {
                          frame False {
                            n722 = local read "estadoTorreTres"() -> (w1099:i32[])
                            n723 = Search 1D Array(1D array=w1099, element=0) -> (index of element=w1098:i32)  [unwired: 1 in]
                            n724 = Equal?(x=w1098, y=-1) -> (x = y?=w1100:bool)
                            n725 = case shown="False" w1100 {
                              tunnel: w1099 -> [w1101 w1112]
                              tunnel: w1098 -> [w1102 _]
                              frame False {
                                n726 = Equal?(x=w1102, y=0) -> (x = y?=w1103:bool)
                                n727 = case shown="False" w1103 {
                                tunnel: w1102 -> [w1109 _]
                                tunnel: w1101 -> [w1107 _]
                                frame False {
                                n728 = Decrement(x=w1109) -> (x-1=w1108:i32)
                                n729 = Replace Array Subset(array=w1107, new element=0 ("new element/subarray"), index=w1108) -> (w1105:i32[])
                                n730 = local write "estadoTorreTres"(w1105) -> ()
                                }
                                frame True {
                                }
                                }
                              }
                              frame True {
                                n731 = Array Size(array=w1112) -> (size(s)=w1114:i32)
                                n732 = Decrement(x=w1114) -> (x-1=w1113:i32)
                                n733 = Replace Array Subset(array=w1112, new element=0 ("new element/subarray"), index=w1113) -> (w1110:i32[])
                                n734 = local write "estadoTorreTres"(w1110) -> ()
                              }
                            }
                          }
                          frame True {
                            n735 = local read "estadoTorreDos"() -> (w1116:i32[])
                            n736 = Search 1D Array(1D array=w1116, element=0) -> (index of element=w1115:i32)  [unwired: 1 in]
                            n737 = Equal?(x=w1115, y=-1) -> (x = y?=w1117:bool)
                            n738 = case shown="True" w1117 {
                              tunnel: w1116 -> [w1120 w1131]
                              tunnel: w1115 -> [w1121 _]
                              frame False {
                                n739 = Equal?(x=w1121, y=0) -> (x = y?=w1122:bool)
                                n740 = case shown="True" w1122 {
                                tunnel: w1121 -> [w1128 _]
                                tunnel: w1120 -> [w1126 _]
                                frame False {
                                n741 = Decrement(x=w1128) -> (x-1=w1127:i32)
                                n742 = Replace Array Subset(array=w1126, new element=0 ("new element/subarray"), index=w1127) -> (w1124:i32[])
                                n743 = local write "estadoTorreDos"(w1124) -> ()
                                }
                                frame True {
                                }
                                }
                              }
                              frame True {
                                n744 = Array Size(array=w1131) -> (size(s)=w1133:i32)
                                n745 = Decrement(x=w1133) -> (x-1=w1132:i32)
                                n746 = Replace Array Subset(array=w1131, new element=0 ("new element/subarray"), index=w1132) -> (w1129:i32[])
                                n747 = local write "estadoTorreDos"(w1129) -> ()
                              }
                            }
                          }
                        }
                      }
                      frame True {
                        n748 = local read "estadoTorreUno"() -> (w1135:i32[])
                        n749 = Search 1D Array(1D array=w1135, element=0) -> (index of element=w1134:i32)  [unwired: 1 in]
                        n750 = Equal?(x=w1134, y=-1) -> (x = y?=w1136:bool)
                        n751 = case shown="False" w1136 {
                          tunnel: w1135 -> [w1139 w1150]
                          tunnel: w1134 -> [w1140 _]
                          frame False {
                            n752 = Equal?(x=w1140, y=0) -> (x = y?=w1141:bool)
                            n753 = case shown="False" w1141 {
                              tunnel: w1140 -> [w1147 _]
                              tunnel: w1139 -> [w1145 _]
                              frame False {
                                n754 = Decrement(x=w1147) -> (x-1=w1146:i32)
                                n755 = Replace Array Subset(array=w1145, new element=0 ("new element/subarray"), index=w1146) -> (w1143:i32[])
                                n756 = local write "estadoTorreUno"(w1143) -> ()
                              }
                              frame True {
                              }
                            }
                          }
                          frame True {
                            n757 = Array Size(array=w1150) -> (size(s)=w1152:i32)
                            n758 = Decrement(x=w1152) -> (x-1=w1151:i32)
                            n759 = Replace Array Subset(array=w1150, new element=0 ("new element/subarray"), index=w1151) -> (w1148:i32[])
                            n760 = local write "estadoTorreUno"(w1148) -> ()
                          }
                        }
                      }
                    }
                    n761 = call "auxiliar.vi"("posicion"=w1079, "numPiezas"=w1088) -> ("posicion"=w1087:i32)
                    n762 = Replace Array Subset(array=w1080, new element=2, index=w1079) -> (w1092:i32[])
                    n763 = Decrement(x=w1087) -> (x-1=w1075:i32)
                    n764 = local write "estadoTorreUno"(w1092) -> ()
                    n765 = local read "posPiezaDos"() -> (w1091:i32[][])
                    n766 = Index Array(array=w1091, index (row) #1=w1075, index (col) #1=0 ("disabled index (col)"), index (row) #2=w1075, index (col) #2=1 ("disabled index (col)")) -> (element #1=w1090:i32, element #2=w1089:i32)
                    n767 = local read "numMov"() -> (w1086:dbl)
                    n768 = Bundle(w1090, w1089) -> (w1081:cluster{i32, i32})  [unwired: 1 in]
                    n769 = Increment(x=w1086) -> (x+1=w1085:dbl)
                    n770 = property on="PiezaDos" class="Bool (strict)"("Position"=w1081) -> ()  [unwired: 2 in, 2 out]
                    n771 = local write "numMov"(w1085) -> ()
                  }
                }
              }
              frame True {
                n772 = local read "numPiezas"() -> (w1166:enum16{"5", "4", "3"})
                n773 = local read "Torre"() -> (w1154:i8)
                n774 = Equal?(x=w1154, y=i8 1) -> (x = y?=w1156:bool)
                n775 = call "auxiliar.vi"("posicion"=w1158, "numPiezas"=w1166) -> ("posicion"=w1165:i32)
                n776 = case shown="False" w1156 {
                  tunnel: w1154 -> [w1171 _]
                  frame False {
                    n777 = Equal?(x=w1171, y=i8 2) -> (x = y?=w1172:bool)
                    n778 = case shown="True" w1172 {
                      frame False {
                        n779 = local read "estadoTorreTres"() -> (w1177:i32[])
                        n780 = Search 1D Array(1D array=w1177, element=0) -> (index of element=w1176:i32)  [unwired: 1 in]
                        n781 = Equal?(x=w1176, y=-1) -> (x = y?=w1178:bool)
                        n782 = case shown="False" w1178 {
                          tunnel: w1177 -> [w1179 w1190]
                          tunnel: w1176 -> [w1180 _]
                          frame False {
                            n783 = Equal?(x=w1180, y=0) -> (x = y?=w1181:bool)
                            n784 = case shown="True" w1181 {
                              tunnel: w1180 -> [w1187 _]
                              tunnel: w1179 -> [w1185 _]
                              frame False {
                                n785 = Decrement(x=w1187) -> (x-1=w1186:i32)
                                n786 = Replace Array Subset(array=w1185, new element=0 ("new element/subarray"), index=w1186) -> (w1183:i32[])
                                n787 = local write "estadoTorreTres"(w1183) -> ()
                              }
                              frame True {
                              }
                            }
                          }
                          frame True {
                            n788 = Array Size(array=w1190) -> (size(s)=w1192:i32)
                            n789 = Decrement(x=w1192) -> (x-1=w1191:i32)
                            n790 = Replace Array Subset(array=w1190, new element=0 ("new element/subarray"), index=w1191) -> (w1188:i32[])
                            n791 = local write "estadoTorreTres"(w1188) -> ()
                          }
                        }
                      }
                      frame True {
                        n792 = local read "estadoTorreDos"() -> (w1194:i32[])
                        n793 = Search 1D Array(1D array=w1194, element=0) -> (index of element=w1193:i32)  [unwired: 1 in]
                        n794 = Equal?(x=w1193, y=-1) -> (x = y?=w1195:bool)
                        n795 = case shown="True" w1195 {
                          tunnel: w1194 -> [w1198 w1209]
                          tunnel: w1193 -> [w1199 _]
                          frame False {
                            n796 = Equal?(x=w1199, y=0) -> (x = y?=w1200:bool)
                            n797 = case shown="True" w1200 {
                              tunnel: w1199 -> [w1206 _]
                              tunnel: w1198 -> [w1204 _]
                              frame False {
                                n798 = Decrement(x=w1206) -> (x-1=w1205:i32)
                                n799 = Replace Array Subset(array=w1204, new element=0 ("new element/subarray"), index=w1205) -> (w1202:i32[])
                                n800 = local write "estadoTorreDos"(w1202) -> ()
                              }
                              frame True {
                              }
                            }
                          }
                          frame True {
                            n801 = Array Size(array=w1209) -> (size(s)=w1211:i32)
                            n802 = Decrement(x=w1211) -> (x-1=w1210:i32)
                            n803 = Replace Array Subset(array=w1209, new element=0 ("new element/subarray"), index=w1210) -> (w1207:i32[])
                            n804 = local write "estadoTorreDos"(w1207) -> ()
                          }
                        }
                      }
                    }
                  }
                  frame True {
                    n805 = local read "estadoTorreUno"() -> (w1213:i32[])
                    n806 = Search 1D Array(1D array=w1213, element=0) -> (index of element=w1212:i32)  [unwired: 1 in]
                    n807 = Equal?(x=w1212, y=-1) -> (x = y?=w1214:bool)
                    n808 = case shown="False" w1214 {
                      tunnel: w1213 -> [w1217 w1228]
                      tunnel: w1212 -> [w1218 _]
                      frame False {
                        n809 = Equal?(x=w1218, y=0) -> (x = y?=w1219:bool)
                        n810 = case shown="False" w1219 {
                          tunnel: w1218 -> [w1225 _]
                          tunnel: w1217 -> [w1223 _]
                          frame False {
                            n811 = Decrement(x=w1225) -> (x-1=w1224:i32)
                            n812 = Replace Array Subset(array=w1223, new element=0 ("new element/subarray"), index=w1224) -> (w1221:i32[])
                            n813 = local write "estadoTorreUno"(w1221) -> ()
                          }
                          frame True {
                          }
                        }
                      }
                      frame True {
                        n814 = Array Size(array=w1228) -> (size(s)=w1230:i32)
                        n815 = Decrement(x=w1230) -> (x-1=w1229:i32)
                        n816 = Replace Array Subset(array=w1228, new element=0 ("new element/subarray"), index=w1229) -> (w1226:i32[])
                        n817 = local write "estadoTorreUno"(w1226) -> ()
                      }
                    }
                  }
                }
                n818 = Replace Array Subset(array=w1157, new element=2, index=w1158) -> (w1170:i32[])
                n819 = Decrement(x=w1165) -> (x-1=w1153:i32)
                n820 = local read "posPiezaDos"() -> (w1169:i32[][])
                n821 = local write "estadoTorreTres"(w1170) -> ()
                n822 = Index Array(array=w1169, index (row) #1=w1153, index (col) #1=4 ("disabled index (col)"), index (row) #2=w1153, index (col) #2=5 ("disabled index (col)")) -> (element #1=w1168:i32, element #2=w1167:i32)
                n823 = local read "numMov"() -> (w1164:dbl)
                n824 = Bundle(w1168, w1167) -> (w1159:cluster{i32, i32})  [unwired: 1 in]
                n825 = Increment(x=w1164) -> (x+1=w1163:dbl)
                n826 = property on="PiezaDos" class="Bool (strict)"("Position"=w1159) -> ()  [unwired: 2 in, 2 out]
                n827 = local write "numMov"(w1163) -> ()
              }
            }
          }
          frame True {
            n828 = local read "numPiezas"() -> (w1244:enum16{"5", "4", "3"})
            n829 = local read "Torre"() -> (w1233:i8)
            n830 = Equal?(x=w1233, y=i8 1) -> (x = y?=w1235:bool)
            n831 = call "auxiliar.vi"("posicion"=w1237, "numPiezas"=w1244) -> ("posicion"=w1243:i32)
            n832 = case shown="False" w1235 {
              tunnel: w1233 -> [w1249 _]
              frame False {
                n833 = Equal?(x=w1249, y=i8 2) -> (x = y?=w1250:bool)
                n834 = case shown="False" w1250 {
                  frame False {
                    n835 = local read "estadoTorreTres"() -> (w1255:i32[])
                    n836 = Search 1D Array(1D array=w1255, element=0) -> (index of element=w1254:i32)  [unwired: 1 in]
                    n837 = Equal?(x=w1254, y=-1) -> (x = y?=w1256:bool)
                    n838 = case shown="False" w1256 {
                      tunnel: w1255 -> [w1257 w1268]
                      tunnel: w1254 -> [w1258 _]
                      frame False {
                        n839 = Equal?(x=w1258, y=0) -> (x = y?=w1259:bool)
                        n840 = case shown="False" w1259 {
                          tunnel: w1258 -> [w1265 _]
                          tunnel: w1257 -> [w1263 _]
                          frame False {
                            n841 = Decrement(x=w1265) -> (x-1=w1264:i32)
                            n842 = Replace Array Subset(array=w1263, new element=0 ("new element/subarray"), index=w1264) -> (w1261:i32[])
                            n843 = local write "estadoTorreTres"(w1261) -> ()
                          }
                          frame True {
                          }
                        }
                      }
                      frame True {
                        n844 = Array Size(array=w1268) -> (size(s)=w1270:i32)
                        n845 = Decrement(x=w1270) -> (x-1=w1269:i32)
                        n846 = Replace Array Subset(array=w1268, new element=0 ("new element/subarray"), index=w1269) -> (w1266:i32[])
                        n847 = local write "estadoTorreTres"(w1266) -> ()
                      }
                    }
                  }
                  frame True {
                    n848 = local read "estadoTorreDos"() -> (w1272:i32[])
                    n849 = Search 1D Array(1D array=w1272, element=0) -> (index of element=w1271:i32)  [unwired: 1 in]
                    n850 = Equal?(x=w1271, y=-1) -> (x = y?=w1273:bool)
                    n851 = case shown="True" w1273 {
                      tunnel: w1272 -> [w1276 w1287]
                      tunnel: w1271 -> [w1277 _]
                      frame False {
                        n852 = Equal?(x=w1277, y=0) -> (x = y?=w1278:bool)
                        n853 = case shown="True" w1278 {
                          tunnel: w1277 -> [w1284 _]
                          tunnel: w1276 -> [w1282 _]
                          frame False {
                            n854 = Decrement(x=w1284) -> (x-1=w1283:i32)
                            n855 = Replace Array Subset(array=w1282, new element=0 ("new element/subarray"), index=w1283) -> (w1280:i32[])
                            n856 = local write "estadoTorreDos"(w1280) -> ()
                          }
                          frame True {
                          }
                        }
                      }
                      frame True {
                        n857 = Array Size(array=w1287) -> (size(s)=w1289:i32)
                        n858 = Decrement(x=w1289) -> (x-1=w1288:i32)
                        n859 = Replace Array Subset(array=w1287, new element=0 ("new element/subarray"), index=w1288) -> (w1285:i32[])
                        n860 = local write "estadoTorreDos"(w1285) -> ()
                      }
                    }
                  }
                }
              }
              frame True {
                n861 = local read "estadoTorreUno"() -> (w1291:i32[])
                n862 = Search 1D Array(1D array=w1291, element=0) -> (index of element=w1290:i32)  [unwired: 1 in]
                n863 = Equal?(x=w1290, y=-1) -> (x = y?=w1292:bool)
                n864 = case shown="False" w1292 {
                  tunnel: w1291 -> [w1295 w1306]
                  tunnel: w1290 -> [w1296 _]
                  frame False {
                    n865 = Equal?(x=w1296, y=0) -> (x = y?=w1297:bool)
                    n866 = case shown="False" w1297 {
                      tunnel: w1296 -> [w1303 _]
                      tunnel: w1295 -> [w1301 _]
                      frame False {
                        n867 = Decrement(x=w1303) -> (x-1=w1302:i32)
                        n868 = Replace Array Subset(array=w1301, new element=0 ("new element/subarray"), index=w1302) -> (w1299:i32[])
                        n869 = local write "estadoTorreUno"(w1299) -> ()
                      }
                      frame True {
                      }
                    }
                  }
                  frame True {
                    n870 = Array Size(array=w1306) -> (size(s)=w1308:i32)
                    n871 = Decrement(x=w1308) -> (x-1=w1307:i32)
                    n872 = Replace Array Subset(array=w1306, new element=0 ("new element/subarray"), index=w1307) -> (w1304:i32[])
                    n873 = local write "estadoTorreUno"(w1304) -> ()
                  }
                }
              }
            }
            n874 = Replace Array Subset(array=w1236, new element=2, index=w1237) -> (w1248:i32[])
            n875 = Decrement(x=w1243) -> (x-1=w1231:i32)
            n876 = local write "estadoTorreDos"(w1248) -> ()
            n877 = local read "posPiezaDos"() -> (w1247:i32[][])
            n878 = Index Array(array=w1247, index (row) #1=w1231, index (col) #1=2 ("disabled index (col)"), index (row) #2=w1231, index (col) #2=3 ("disabled index (col)")) -> (element #1=w1246:i32, element #2=w1245:i32)
            n879 = local read "numMov"() -> (w1242:dbl)
            n880 = Bundle(w1246, w1245) -> (w1232:cluster{i32, i32})  [unwired: 1 in]
            n881 = Increment(x=w1242) -> (x+1=w1241:dbl)
            n882 = property on="PiezaDos" class="Bool (strict)"("Position"=w1232) -> ()  [unwired: 2 in, 2 out]
            n883 = local write "numMov"(w1241) -> ()
          }
        }
      }
      event "PiezaTres": Mouse Down {
        n884 = event-data() -> ()  [unwired: 1 in, 1 out]
        n885 = property on="PiezaTres" class="Bool (strict)"() -> ("Position"=w1313:T1)  [unwired: 2 in, 2 out]
        "PosAntPiezaTres" <- w1313
        n886 = local write "¿Pieza?"(i8 3 ("¿Pieza?")) -> ()
        n887 = Cluster To Array(cluster=w1313) -> (array=w1315:i32[])
        n888 = local read "posPiezaTres"() -> (w1314:i32[][])
        n889 = call "direccionPieza.vi"("posicion"=w1315, "matrizPosiciones"=w1314) -> ("Posicion"=w1311:i32, "Torre"=w1312:i8)
        n890 = local write "Torre"(w1312) -> ()
        n891 = Add(x=w1311, y=2) -> (x+y=w1309:i32)
        n892 = local write "Posicion"(w1309) -> ()
      }
      event "PiezaTres": Mouse Up {
        n893 = event-data() -> ("Coords"=w1328:T4)  [unwired: 1 in]
        n894 = property on="TorreUno" class="Slide (strict)"() -> ("Position"=w1344:T1, "Left"=w1346:i32, "Top"=w1349:i32, "Bounds"=w1343:T3, "Height"=w1348:u32, "Width"=w1338:u32)  [unwired: 2 in, 2 out]
        n895 = property on="TorreTres" class="Slide (strict)"() -> ("Position"=w1353:T1, "Left"=w1356:i32, "Top"=w1359:i32, "Bounds"=w1354:T3, "Height"=w1358:u32, "Width"=w1362:u32)  [unwired: 2 in, 2 out]
        n896 = property on="TorreDos" class="Slide (strict)"() -> ("Position"=w1368:T1, "Left"=w1364:i32, "Top"=w1366:i32, "Bounds"=w1369:T3, "Height"=w1365:u32, "Width"=w1340:u32)  [unwired: 2 in, 2 out]
        n897 = local read "estadoTorreTres"() -> (w1322:i32[])
        n898 = local read "estadoTorreDos"() -> (w1325:i32[])
        n899 = local read "estadoTorreUno"() -> (w1319:i32[])
        n900 = local read "¿Pieza?"() -> (w1336:i8)
        n901 = local read "¿Pieza?"() -> (w1337:i8)
        n902 = local read "¿Pieza?"() -> (w1335:i8)
        n903 = Add(x=w1346, y=w1338) -> (x+y=w1350:u32)
        n904 = Add(x=w1349, y=w1348) -> (x+y=w1347:u32)
        n905 = Add(x=w1344, y=w1343) -> (x+y=w1342:T3)
        n906 = Add(x=w1356, y=w1362) -> (x+y=w1361:u32)
        n907 = Add(x=w1353, y=w1354) -> (x+y=w1352:T3)
        n908 = Add(x=w1359, y=w1358) -> (x+y=w1357:u32)
        n909 = Add(x=w1364, y=w1340) -> (x+y=w1370:u32)
        n910 = Add(x=w1368, y=w1369) -> (x+y=w1367:T3)
        n911 = Add(x=w1366, y=w1365) -> (x+y=w1363:u32)
        n912 = call "estadoTorre.vi"("¿pieza?"=w1336, "estadoTorre"=w1322) -> ("¿disponible?"=w1331:bool, "posicionCero"=w1323:i32)
        n913 = call "estadoTorre.vi"("¿pieza?"=w1337, "estadoTorre"=w1325) -> ("¿disponible?"=w1333:bool, "posicionCero"=w1326:i32)
        n914 = call "estadoTorre.vi"("¿pieza?"=w1335, "estadoTorre"=w1319) -> ("¿disponible?"=w1329:bool, "posicionCero"=w1320:i32)
        n915 = Bundle(w1350, "Top"=w1349) -> (w1351:cluster{u32, "Top":i32})  [unwired: 1 in]
        n916 = Bundle("Left"=w1346, w1347) -> (w1345:cluster{"Left":i32, u32})  [unwired: 1 in]
        n917 = Bundle(w1361, "Top"=w1359) -> (w1360:cluster{u32, "Top":i32})  [unwired: 1 in]
        n918 = Bundle("Left"=w1356, w1357) -> (w1355:cluster{"Left":i32, u32})  [unwired: 1 in]
        n919 = Bundle(w1370, "Top"=w1366) -> (w1339:cluster{u32, "Top":i32})  [unwired: 1 in]
        n920 = Bundle("Left"=w1364, w1363) -> (w1341:cluster{"Left":i32, u32})  [unwired: 1 in]
        n921 = call "perteneceAtorre.vi"("P1"=w1344, "P2"=w1351, "P"=w1328, "P3"=w1345, "P4"=w1342) -> ("out"=w1330:bool)
        n922 = call "perteneceAtorre.vi"("P1"=w1353, "P2"=w1360, "P"=w1328, "P3"=w1352, "P4"=w1355) -> ("out"=w1332:bool)
        n923 = call "perteneceAtorre.vi"("P1"=w1368, "P2"=w1339, "P"=w1328, "P3"=w1367, "P4"=w1341) -> ("out"=w1334:bool)
        n924 = And(x=w1330, y=w1329) -> (x .and. y?=w1321:bool)
        n925 = And(x=w1334, y=w1333) -> (x .and. y?=w1327:bool)
        n926 = And(x=w1332, y=w1331) -> (x .and. y?=w1324:bool)
        n927 = case shown="True" w1327 {
          tunnel: w1326 -> [_ w1610]
          tunnel: w1325 -> [_ w1611]
          tunnel: w1324 -> [w1378 _]
          tunnel: w1323 -> [w1377 _]
          tunnel: w1322 -> [w1376 _]
          tunnel: w1321 -> [w1375 _]
          tunnel: w1320 -> [w1374 _]
          tunnel: w1319 -> [w1373 _]
          frame False {
            n928 = case shown="True" w1378 {
              tunnel: w1377 -> [_ w1532]
              tunnel: w1376 -> [_ w1533]
              tunnel: w1375 -> [w1381 _]
              tunnel: w1374 -> [w1380 _]
              tunnel: w1373 -> [w1379 _]
              frame False {
                n929 = case shown="True" w1381 {
                  tunnel: w1380 -> [_ w1391]
                  tunnel: w1379 -> [_ w1390]
                  frame False {
                    n930 = local read "PosAntPiezaTres"() -> (w1382:T1)
                    n931 = property on="PiezaTres" class="Bool (strict)"("Position"=w1382) -> ()  [unwired: 2 in, 2 out]
                  }
                  frame True {
                    n932 = local read "numPiezas"() -> (w1400:enum16{"5", "4", "3"})
                    n933 = call "auxiliar.vi"("posicion"=w1391, "numPiezas"=w1400) -> ("posicion"=w1399:i32)
                    n934 = Replace Array Subset(array=w1390, new element=3, index=w1391) -> (w1404:i32[])
                    n935 = Decrement(x=w1399) -> (x-1=w1393:i32)
                    n936 = local read "Torre"() -> (w1389:i8)
                    n937 = local read "Torre"() -> (w1384:i8)
                    n938 = local read "posPiezaTres"() -> (w1403:i32[][])
                    n939 = local write "estadoTorreTres"(w1404) -> ()
                    n940 = Decrement(x=w1393) -> (x-1=w1383:i32)
                    n941 = Equal?(x=w1389, y=i8 1) -> (x = y?=w1387:bool)
                    n942 = Equal?(x=w1384, y=i8 1) -> (x = y?=w1386:bool)
                    n943 = case shown="False" w1387 {
                      tunnel: w1389 -> [w1405 _]
                      frame False {
                        n944 = Equal?(x=w1405, y=i8 2) -> (x = y?=w1406:bool)
                        n945 = case shown="False" w1406 {
                          frame False {
                            n946 = local read "estadoTorreTres"() -> (w1411:i32[])
                            n947 = Search 1D Array(1D array=w1411, element=0) -> (index of element=w1410:i32)  [unwired: 1 in]
                            n948 = Equal?(x=w1410, y=-1) -> (x = y?=w1412:bool)
                            n949 = case shown="False" w1412 {
                              tunnel: w1411 -> [w1413 w1424]
                              tunnel: w1410 -> [w1414 _]
                              frame False {
                                n950 = Equal?(x=w1414, y=0) -> (x = y?=w1415:bool)
                                n951 = case shown="False" w1415 {
                                tunnel: w1414 -> [w1421 _]
                                tunnel: w1413 -> [w1419 _]
                                frame False {
                                n952 = Decrement(x=w1421) -> (x-1=w1420:i32)
                                n953 = Replace Array Subset(array=w1419, new element=0 ("new element/subarray"), index=w1420) -> (w1417:i32[])
                                n954 = local write "estadoTorreTres"(w1417) -> ()
                                }
                                frame True {
                                }
                                }
                              }
                              frame True {
                                n955 = Array Size(array=w1424) -> (size(s)=w1426:i32)
                                n956 = Decrement(x=w1426) -> (x-1=w1425:i32)
                                n957 = Replace Array Subset(array=w1424, new element=0 ("new element/subarray"), index=w1425) -> (w1422:i32[])
                                n958 = local write "estadoTorreTres"(w1422) -> ()
                              }
                            }
                          }
                          frame True {
                            n959 = local read "estadoTorreDos"() -> (w1428:i32[])
                            n960 = Search 1D Array(1D array=w1428, element=0) -> (index of element=w1427:i32)  [unwired: 1 in]
                            n961 = Equal?(x=w1427, y=-1) -> (x = y?=w1429:bool)
                            n962 = case shown="True" w1429 {
                              tunnel: w1428 -> [w1432 w1443]
                              tunnel: w1427 -> [w1433 _]
                              frame False {
                                n963 = Equal?(x=w1433, y=0) -> (x = y?=w1434:bool)
                                n964 = case shown="True" w1434 {
                                tunnel: w1433 -> [w1440 _]
                                tunnel: w1432 -> [w1438 _]
                                frame False {
                                n965 = Decrement(x=w1440) -> (x-1=w1439:i32)
                                n966 = Replace Array Subset(array=w1438, new element=0 ("new element/subarray"), index=w1439) -> (w1436:i32[])
                                n967 = local write "estadoTorreDos"(w1436) -> ()
                                }
                                frame True {
                                }
                                }
                              }
                              frame True {
                                n968 = Array Size(array=w1443) -> (size(s)=w1445:i32)
                                n969 = Decrement(x=w1445) -> (x-1=w1444:i32)
                                n970 = Replace Array Subset(array=w1443, new element=0 ("new element/subarray"), index=w1444) -> (w1441:i32[])
                                n971 = local write "estadoTorreDos"(w1441) -> ()
                              }
                            }
                          }
                        }
                      }
                      frame True {
                        n972 = local read "estadoTorreUno"() -> (w1447:i32[])
                        n973 = Search 1D Array(1D array=w1447, element=0) -> (index of element=w1446:i32)  [unwired: 1 in]
                        n974 = Equal?(x=w1446, y=-1) -> (x = y?=w1448:bool)
                        n975 = case shown="False" w1448 {
                          tunnel: w1447 -> [w1451 w1462]
                          tunnel: w1446 -> [w1452 _]
                          frame False {
                            n976 = Equal?(x=w1452, y=0) -> (x = y?=w1453:bool)
                            n977 = case shown="False" w1453 {
                              tunnel: w1452 -> [w1459 _]
                              tunnel: w1451 -> [w1457 _]
                              frame False {
                                n978 = Decrement(x=w1459) -> (x-1=w1458:i32)
                                n979 = Replace Array Subset(array=w1457, new element=0 ("new element/subarray"), index=w1458) -> (w1455:i32[])
                                n980 = local write "estadoTorreUno"(w1455) -> ()
                              }
                              frame True {
                              }
                            }
                          }
                          frame True {
                            n981 = Array Size(array=w1462) -> (size(s)=w1464:i32)
                            n982 = Decrement(x=w1464) -> (x-1=w1463:i32)
                            n983 = Replace Array Subset(array=w1462, new element=0 ("new element/subarray"), index=w1463) -> (w1460:i32[])
                            n984 = local write "estadoTorreUno"(w1460) -> ()
                          }
                        }
                      }
                    }
                    n985 = case shown="False" w1386 {
                      tunnel: w1384 -> [w1465 _]
                      frame False {
                        n986 = Equal?(x=w1465, y=i8 2) -> (x = y?=w1466:bool)
                        n987 = case shown="False" w1466 {
                          frame False {
                            n988 = local read "estadoTorreTres"() -> (w1471:i32[])
                            n989 = Search 1D Array(1D array=w1471, element=0) -> (index of element=w1470:i32)  [unwired: 1 in]
                            n990 = Equal?(x=w1470, y=-1) -> (x = y?=w1472:bool)
                            n991 = case shown="False" w1472 {
                              tunnel: w1471 -> [w1473 w1484]
                              tunnel: w1470 -> [w1474 _]
                              frame False {
                                n992 = Equal?(x=w1474, y=0) -> (x = y?=w1475:bool)
                                n993 = case shown="False" w1475 {
                                tunnel: w1474 -> [w1481 _]
                                tunnel: w1473 -> [w1479 _]
                                frame False {
                                n994 = Decrement(x=w1481) -> (x-1=w1480:i32)
                                n995 = Replace Array Subset(array=w1479, new element=0 ("new element/subarray"), index=w1480) -> (w1477:i32[])
                                n996 = local write "estadoTorreTres"(w1477) -> ()
                                }
                                frame True {
                                }
                                }
                              }
                              frame True {
                                n997 = Array Size(array=w1484) -> (size(s)=w1486:i32)
                                n998 = Decrement(x=w1486) -> (x-1=w1485:i32)
                                n999 = Replace Array Subset(array=w1484, new element=0 ("new element/subarray"), index=w1485) -> (w1482:i32[])
                                n1000 = local write "estadoTorreTres"(w1482) -> ()
                              }
                            }
                          }
                          frame True {
                            n1001 = local read "estadoTorreDos"() -> (w1488:i32[])
                            n1002 = Search 1D Array(1D array=w1488, element=0) -> (index of element=w1487:i32)  [unwired: 1 in]
                            n1003 = Equal?(x=w1487, y=-1) -> (x = y?=w1489:bool)
                            n1004 = case shown="True" w1489 {
                              tunnel: w1488 -> [w1492 w1503]
                              tunnel: w1487 -> [w1493 _]
                              frame False {
                                n1005 = Equal?(x=w1493, y=0) -> (x = y?=w1494:bool)
                                n1006 = case shown="True" w1494 {
                                tunnel: w1493 -> [w1500 _]
                                tunnel: w1492 -> [w1498 _]
                                frame False {
                                n1007 = Decrement(x=w1500) -> (x-1=w1499:i32)
                                n1008 = Replace Array Subset(array=w1498, new element=0 ("new element/subarray"), index=w1499) -> (w1496:i32[])
                                n1009 = local write "estadoTorreDos"(w1496) -> ()
                                }
                                frame True {
                                }
                                }
                              }
                              frame True {
                                n1010 = Array Size(array=w1503) -> (size(s)=w1505:i32)
                                n1011 = Decrement(x=w1505) -> (x-1=w1504:i32)
                                n1012 = Replace Array Subset(array=w1503, new element=0 ("new element/subarray"), index=w1504) -> (w1501:i32[])
                                n1013 = local write "estadoTorreDos"(w1501) -> ()
                              }
                            }
                          }
                        }
                      }
                      frame True {
                        n1014 = local read "estadoTorreUno"() -> (w1507:i32[])
                        n1015 = Search 1D Array(1D array=w1507, element=0) -> (index of element=w1506:i32)  [unwired: 1 in]
                        n1016 = Equal?(x=w1506, y=-1) -> (x = y?=w1508:bool)
                        n1017 = case shown="False" w1508 {
                          tunnel: w1507 -> [w1511 w1522]
                          tunnel: w1506 -> [w1512 _]
                          frame False {
                            n1018 = Equal?(x=w1512, y=0) -> (x = y?=w1513:bool)
                            n1019 = case shown="False" w1513 {
                              tunnel: w1512 -> [w1519 _]
                              tunnel: w1511 -> [w1517 _]
                              frame False {
                                n1020 = Decrement(x=w1519) -> (x-1=w1518:i32)
                                n1021 = Replace Array Subset(array=w1517, new element=0 ("new element/subarray"), index=w1518) -> (w1515:i32[])
                                n1022 = local write "estadoTorreUno"(w1515) -> ()
                              }
                              frame True {
                              }
                            }
                          }
                          frame True {
                            n1023 = Array Size(array=w1522) -> (size(s)=w1524:i32)
                            n1024 = Decrement(x=w1524) -> (x-1=w1523:i32)
                            n1025 = Replace Array Subset(array=w1522, new element=0 ("new element/subarray"), index=w1523) -> (w1520:i32[])
                            n1026 = local write "estadoTorreUno"(w1520) -> ()
                          }
                        }
                      }
                    }
                    n1027 = Index Array(array=w1403, index (row) #1=w1383, index (col) #1=0 ("disabled index (col)"), index (row) #2=w1383, index (col) #2=1 ("disabled index (col)")) -> (element #1=w1402:i32, element #2=w1401:i32)
                    n1028 = local read "numMov"() -> (w1398:dbl)
                    n1029 = Bundle(w1402, w1401) -> (w1392:cluster{i32, i32})  [unwired: 1 in]
                    n1030 = Increment(x=w1398) -> (x+1=w1397:dbl)
                    n1031 = property on="PiezaTres" class="Bool (strict)"("Position"=w1392) -> ()  [unwired: 2 in, 2 out]
                    n1032 = local write "numMov"(w1397) -> ()
                  }
                }
              }
              frame True {
                n1033 = local read "Torre"() -> (w1526:i8)
                n1034 = local read "Torre"() -> (w1530:i8)
                n1035 = local read "numPiezas"() -> (w1541:enum16{"5", "4", "3"})
                n1036 = Equal?(x=w1530, y=i8 1) -> ()  [unwired: 1 out]
                n1037 = Equal?(x=w1526, y=i8 1) -> (x = y?=w1528:bool)
                n1038 = case shown="False" w1528 {
                  tunnel: w1526 -> [w1546 _]
                  frame False {
                    n1039 = Equal?(x=w1546, y=i8 2) -> (x = y?=w1547:bool)
                    n1040 = case shown="False" w1547 {
                      frame False {
                        n1041 = local read "estadoTorreTres"() -> (w1552:i32[])
                        n1042 = Search 1D Array(1D array=w1552, element=0) -> (index of element=w1551:i32)  [unwired: 1 in]
                        n1043 = Equal?(x=w1551, y=-1) -> (x = y?=w1553:bool)
                        n1044 = case shown="False" w1553 {
                          tunnel: w1552 -> [w1554 w1565]
                          tunnel: w1551 -> [w1555 _]
                          frame False {
                            n1045 = Equal?(x=w1555, y=0) -> (x = y?=w1556:bool)
                            n1046 = case shown="False" w1556 {
                              tunnel: w1555 -> [w1562 _]
                              tunnel: w1554 -> [w1560 _]
                              frame False {
                                n1047 = Decrement(x=w1562) -> (x-1=w1561:i32)
                                n1048 = Replace Array Subset(array=w1560, new element=0 ("new element/subarray"), index=w1561) -> (w1558:i32[])
                                n1049 = local write "estadoTorreTres"(w1558) -> ()
                              }
                              frame True {
                              }
                            }
                          }
                          frame True {
                            n1050 = Array Size(array=w1565) -> (size(s)=w1567:i32)
                            n1051 = Decrement(x=w1567) -> (x-1=w1566:i32)
                            n1052 = Replace Array Subset(array=w1565, new element=0 ("new element/subarray"), index=w1566) -> (w1563:i32[])
                            n1053 = local write "estadoTorreTres"(w1563) -> ()
                          }
                        }
                      }
                      frame True {
                        n1054 = local read "estadoTorreDos"() -> (w1569:i32[])
                        n1055 = Search 1D Array(1D array=w1569, element=0) -> (index of element=w1568:i32)  [unwired: 1 in]
                        n1056 = Equal?(x=w1568, y=-1) -> (x = y?=w1570:bool)
                        n1057 = case shown="True" w1570 {
                          tunnel: w1569 -> [w1573 w1584]
                          tunnel: w1568 -> [w1574 _]
                          frame False {
                            n1058 = Equal?(x=w1574, y=0) -> (x = y?=w1575:bool)
                            n1059 = case shown="True" w1575 {
                              tunnel: w1574 -> [w1581 _]
                              tunnel: w1573 -> [w1579 _]
                              frame False {
                                n1060 = Decrement(x=w1581) -> (x-1=w1580:i32)
                                n1061 = Replace Array Subset(array=w1579, new element=0 ("new element/subarray"), index=w1580) -> (w1577:i32[])
                                n1062 = local write "estadoTorreDos"(w1577) -> ()
                              }
                              frame True {
                              }
                            }
                          }
                          frame True {
                            n1063 = Array Size(array=w1584) -> (size(s)=w1586:i32)
                            n1064 = Decrement(x=w1586) -> (x-1=w1585:i32)
                            n1065 = Replace Array Subset(array=w1584, new element=0 ("new element/subarray"), index=w1585) -> (w1582:i32[])
                            n1066 = local write "estadoTorreDos"(w1582) -> ()
                          }
                        }
                      }
                    }
                  }
                  frame True {
                    n1067 = local read "estadoTorreUno"() -> (w1588:i32[])
                    n1068 = Search 1D Array(1D array=w1588, element=0) -> (index of element=w1587:i32)  [unwired: 1 in]
                    n1069 = Equal?(x=w1587, y=-1) -> (x = y?=w1589:bool)
                    n1070 = case shown="False" w1589 {
                      tunnel: w1588 -> [w1592 w1603]
                      tunnel: w1587 -> [w1593 _]
                      frame False {
                        n1071 = Equal?(x=w1593, y=0) -> (x = y?=w1594:bool)
                        n1072 = case shown="False" w1594 {
                          tunnel: w1593 -> [w1600 _]
                          tunnel: w1592 -> [w1598 _]
                          frame False {
                            n1073 = Decrement(x=w1600) -> (x-1=w1599:i32)
                            n1074 = Replace Array Subset(array=w1598, new element=0 ("new element/subarray"), index=w1599) -> (w1596:i32[])
                            n1075 = local write "estadoTorreUno"(w1596) -> ()
                          }
                          frame True {
                          }
                        }
                      }
                      frame True {
                        n1076 = Array Size(array=w1603) -> (size(s)=w1605:i32)
                        n1077 = Decrement(x=w1605) -> (x-1=w1604:i32)
                        n1078 = Replace Array Subset(array=w1603, new element=0 ("new element/subarray"), index=w1604) -> (w1601:i32[])
                        n1079 = local write "estadoTorreUno"(w1601) -> ()
                      }
                    }
                  }
                }
                n1080 = call "auxiliar.vi"("posicion"=w1532, "numPiezas"=w1541) -> ("posicion"=w1540:i32)
                n1081 = Replace Array Subset(array=w1533, new element=3, index=w1532) -> (w1545:i32[])
                n1082 = Decrement(x=w1540) -> (x-1=w1534:i32)
                n1083 = local read "posPiezaTres"() -> (w1544:i32[][])
                n1084 = local write "estadoTorreTres"(w1545) -> ()
                n1085 = Decrement(x=w1534) -> (x-1=w1525:i32)
                n1086 = Index Array(array=w1544, index (row) #1=w1525, index (col) #1=4 ("disabled index (col)"), index (row) #2=w1525, index (col) #2=5 ("disabled index (col)")) -> (element #1=w1543:i32, element #2=w1542:i32)
                n1087 = local read "numMov"() -> (w1539:dbl)
                n1088 = Bundle(w1543, w1542) -> (w1531:cluster{i32, i32})  [unwired: 1 in]
                n1089 = Increment(x=w1539) -> (x+1=w1538:dbl)
                n1090 = property on="PiezaTres" class="Bool (strict)"("Position"=w1531) -> ()  [unwired: 2 in, 2 out]
                n1091 = local write "numMov"(w1538) -> ()
              }
            }
          }
          frame True {
            n1092 = local read "numPiezas"() -> (w1620:enum16{"5", "4", "3"})
            n1093 = local read "Torre"() -> (w1609:i8)
            n1094 = call "auxiliar.vi"("posicion"=w1610, "numPiezas"=w1620) -> ("posicion"=w1619:i32)
            n1095 = Replace Array Subset(array=w1611, new element=3, index=w1610) -> (w1624:i32[])
            n1096 = Decrement(x=w1619) -> (x-1=w1613:i32)
            n1097 = Equal?(x=w1609, y=i8 1) -> (x = y?=w1607:bool)
            n1098 = local read "posPiezaTres"() -> (w1623:i32[][])
            n1099 = local write "estadoTorreTres"(w1624) -> ()
            n1100 = case shown="True" w1607 {
              tunnel: w1609 -> [w1625 _]
              frame False {
                n1101 = Equal?(x=w1625, y=i8 2) -> (x = y?=w1626:bool)
                n1102 = case shown="False" w1626 {
                  frame False {
                    n1103 = local read "estadoTorreTres"() -> (w1631:i32[])
                    n1104 = Search 1D Array(1D array=w1631, element=0) -> (index of element=w1630:i32)  [unwired: 1 in]
                    n1105 = Equal?(x=w1630, y=-1) -> (x = y?=w1632:bool)
                    n1106 = case shown="False" w1632 {
                      tunnel: w1631 -> [w1633 w1644]
                      tunnel: w1630 -> [w1634 _]
                      frame False {
                        n1107 = Equal?(x=w1634, y=0) -> (x = y?=w1635:bool)
                        n1108 = case shown="False" w1635 {
                          tunnel: w1634 -> [w1641 _]
                          tunnel: w1633 -> [w1639 _]
                          frame False {
                            n1109 = Decrement(x=w1641) -> (x-1=w1640:i32)
                            n1110 = Replace Array Subset(array=w1639, new element=0 ("new element/subarray"), index=w1640) -> (w1637:i32[])
                            n1111 = local write "estadoTorreTres"(w1637) -> ()
                          }
                          frame True {
                          }
                        }
                      }
                      frame True {
                        n1112 = Array Size(array=w1644) -> (size(s)=w1646:i32)
                        n1113 = Decrement(x=w1646) -> (x-1=w1645:i32)
                        n1114 = Replace Array Subset(array=w1644, new element=0 ("new element/subarray"), index=w1645) -> (w1642:i32[])
                        n1115 = local write "estadoTorreTres"(w1642) -> ()
                      }
                    }
                  }
                  frame True {
                    n1116 = local read "estadoTorreDos"() -> (w1648:i32[])
                    n1117 = Search 1D Array(1D array=w1648, element=0) -> (index of element=w1647:i32)  [unwired: 1 in]
                    n1118 = Equal?(x=w1647, y=-1) -> (x = y?=w1649:bool)
                    n1119 = case shown="True" w1649 {
                      tunnel: w1648 -> [w1652 w1663]
                      tunnel: w1647 -> [w1653 _]
                      frame False {
                        n1120 = Equal?(x=w1653, y=0) -> (x = y?=w1654:bool)
                        n1121 = case shown="True" w1654 {
                          tunnel: w1653 -> [w1660 _]
                          tunnel: w1652 -> [w1658 _]
                          frame False {
                            n1122 = Decrement(x=w1660) -> (x-1=w1659:i32)
                            n1123 = Replace Array Subset(array=w1658, new element=0 ("new element/subarray"), index=w1659) -> (w1656:i32[])
                            n1124 = local write "estadoTorreDos"(w1656) -> ()
                          }
                          frame True {
                          }
                        }
                      }
                      frame True {
                        n1125 = Array Size(array=w1663) -> (size(s)=w1665:i32)
                        n1126 = Decrement(x=w1665) -> (x-1=w1664:i32)
                        n1127 = Replace Array Subset(array=w1663, new element=0 ("new element/subarray"), index=w1664) -> (w1661:i32[])
                        n1128 = local write "estadoTorreDos"(w1661) -> ()
                      }
                    }
                  }
                }
              }
              frame True {
                n1129 = local read "estadoTorreUno"() -> (w1667:i32[])
                n1130 = Search 1D Array(1D array=w1667, element=0) -> (index of element=w1666:i32)  [unwired: 1 in]
                n1131 = Equal?(x=w1666, y=-1) -> (x = y?=w1668:bool)
                n1132 = case shown="False" w1668 {
                  tunnel: w1667 -> [w1671 w1682]
                  tunnel: w1666 -> [w1672 _]
                  frame False {
                    n1133 = Equal?(x=w1672, y=0) -> (x = y?=w1673:bool)
                    n1134 = case shown="False" w1673 {
                      tunnel: w1672 -> [w1679 _]
                      tunnel: w1671 -> [w1677 _]
                      frame False {
                        n1135 = Decrement(x=w1679) -> (x-1=w1678:i32)
                        n1136 = Replace Array Subset(array=w1677, new element=0 ("new element/subarray"), index=w1678) -> (w1675:i32[])
                        n1137 = local write "estadoTorreUno"(w1675) -> ()
                      }
                      frame True {
                      }
                    }
                  }
                  frame True {
                    n1138 = Array Size(array=w1682) -> (size(s)=w1684:i32)
                    n1139 = Decrement(x=w1684) -> (x-1=w1683:i32)
                    n1140 = Replace Array Subset(array=w1682, new element=0 ("new element/subarray"), index=w1683) -> (w1680:i32[])
                    n1141 = local write "estadoTorreUno"(w1680) -> ()
                  }
                }
              }
            }
            n1142 = Decrement(x=w1613) -> (x-1=w1606:i32)
            n1143 = Index Array(array=w1623, index (row) #1=w1606, index (col) #1=2 ("disabled index (col)"), index (row) #2=w1606, index (col) #2=3 ("disabled index (col)")) -> (element #1=w1622:i32, element #2=w1621:i32)
            n1144 = local read "numMov"() -> (w1618:dbl)
            n1145 = Bundle(w1622, w1621) -> (w1612:cluster{i32, i32})  [unwired: 1 in]
            n1146 = Increment(x=w1618) -> (x+1=w1617:dbl)
            n1147 = property on="PiezaTres" class="Bool (strict)"("Position"=w1612) -> ()  [unwired: 2 in, 2 out]
            n1148 = local write "numMov"(w1617) -> ()
          }
        }
      }
      event "PiezaCuatro": Mouse Down? {
        n1149 = event-data() -> ()  [unwired: 1 in, 1 out]
        n1150 = property on="PiezaCinco" class="Bool (strict)"() -> ("Position"=w1685:T1)  [unwired: 2 in, 2 out]
        "PosAntPiezaCuatro" <- w1685
        n1151 = local read "posPiezaUno"() -> (w1690:i32[][])
        n1152 = local write "¿Pieza?"(i8 4 ("¿Pieza?")) -> ()
        n1153 = Cluster To Array(cluster=w1685) -> (array=w1691:i32[])
        n1154 = call "direccionPieza.vi"("posicion"=w1691, "matrizPosiciones"=w1690) -> ("Posicion"=w1688:i32, "Torre"=w1689:i8)
        n1155 = local write "Torre"(w1689) -> ()
        n1156 = Add(x=w1688, y=3) -> (x+y=w1686:i32)
        n1157 = local write "Posicion"(w1686) -> ()
        n1158 = event-data("Discard?"=FALSE) -> ()  [unwired: 1 in, 1 out]
      }
      event "PiezaCinco": Mouse Down? {
        n1159 = event-data() -> ()  [unwired: 1 in, 1 out]
        n1160 = property on="PiezaCinco" class="Bool (strict)"() -> ("Position"=w1702:T1)  [unwired: 2 in, 2 out]
        "PosAntPiezaCinco" <- w1702
        n1161 = local read "posPiezaUno"() -> (w1705:i32[][])
        n1162 = Cluster To Array(cluster=w1702) -> (array=w1706:i32[])
        n1163 = local write "¿Pieza?"(i8 5 ("¿Pieza?")) -> ()
        n1164 = call "direccionPieza.vi"("posicion"=w1706, "matrizPosiciones"=w1705) -> ("Posicion"=w1701:i32, "Torre"=w1704:i8)
        n1165 = local write "Torre"(w1704) -> ()
        n1166 = Add(x=w1701, y=4) -> (x+y=w1699:i32)
        n1167 = local write "Posicion"(w1699) -> ()
        n1168 = event-data("Discard?"=FALSE) -> ()  [unwired: 1 in, 1 out]
      }
      event "Iniciar": Value Change {
        n1169 = event-data() -> ()  [unwired: 1 in, 6 out]
        n1170 = case shown="\"4\"" "numPiezas" {
          frame "3", Default {
            w1736 = 0 ("index (row)")
            n1171 = local read "matrizPosIniciales"() -> (w1739:T2)
            n1172 = local write "minMov"(7.0 ("minMov")) -> ()
            n1173 = Index Array(array=w1739, index (row) #1=w1736, index (col) #1=w1736, index (row) #2=w1736, index (col) #2=1 ("disabled index (col)"), index (row) #3=w1736, index (col) #3=2 ("disabled index (col)"), index (row) #4=w1736, index (col) #4=3 ("disabled index (col)"), index (row) #5=w1736, index (col) #5=4 ("disabled index (col)"), index (row) #6=w1736, index (col) #6=5 ("disabled index (col)")) -> (element #1=w1732:dbl, element #2=w1731:dbl, element #3=w1730:dbl, element #4=w1729:dbl, element #5=w1728:dbl, element #6=w1727:dbl)
            n1174 = property on="PiezaUno" class="Bool (strict)"("Left"=w1732, "Top"=w1731) -> ()  [unwired: 2 in, 2 out]
            n1175 = property on="PiezaDos" class="Bool (strict)"("Left"=w1730, "Top"=w1729) -> ()  [unwired: 2 in, 2 out]
            n1176 = property on="PiezaTres" class="Bool (strict)"("Left"=w1728, "Top"=w1727) -> ()  [unwired: 2 in, 2 out]
            n1177 = Initialize Array(0, 3 ("dimension size")) -> (w1717:i32[])
            n1178 = local write "estadoTorreDos"(w1717) -> ()
            n1179 = local write "estadoTorreTres"(w1717) -> ()
            n1180 = Replace Array Subset(array=w1717, new element #1=3 ("new element/subarray"), index #1=0 ("index"), new element #2=2 ("new element/subarray"), index #2=1 ("index"), new element #3=1 ("new element/subarray"), index #3=2 ("index")) -> (w1710:i32[])
            n1181 = local write "estadoTorreUno"(w1710) -> ()
            n1182 = property on="PiezaCinco" class="Bool (strict)"("Visible"=FALSE ("PiezaCinco")) -> ()  [unwired: 2 in, 2 out]
            n1183 = property on="PiezaCuatro" class="Bool (strict)"("Visible"=FALSE ("PiezaCuatro")) -> ()  [unwired: 2 in, 2 out]
            n1184 = property on="PiezaUno" class="Bool (strict)"("Visible"=TRUE) -> ()  [unwired: 2 in, 2 out]
            n1185 = property on="PiezaDos" class="Bool (strict)"("Visible"=TRUE ("PiezaDos")) -> ()  [unwired: 2 in, 2 out]
            n1186 = property on="PiezaTres" class="Bool (strict)"("Visible"=TRUE) -> ()  [unwired: 2 in, 2 out]
            n1187 = property on="PiezaCinco" class="Bool (strict)"("Position"=T1 {"Left"=967, "Top"=119}) -> ()  [unwired: 2 in, 2 out]
            n1188 = property on="PiezaCuatro" class="Bool (strict)"("Position"=T1 {"Left"=995, "Top"=95}) -> ()  [unwired: 2 in, 2 out]
          }
          frame "4" {
            w1773 = 1
            n1189 = local read "matrizPosIniciales"() -> (w1775:T2)
            n1190 = Initialize Array(0, 4 ("dimension size")) -> (w1750:i32[])
            n1191 = local write "estadoTorreDos"(w1750) -> ()
            n1192 = local write "estadoTorreTres"(w1750) -> ()
            n1193 = Replace Array Subset(array=w1750, new element #1=4 ("new element/subarray"), index #1=0 ("index"), new element #2=3 ("new element/subarray"), index #2=1 ("index"), new element #3=2 ("new element/subarray"), index #3=2 ("index"), new element #4=1 ("new element/subarray"), index #4=3 ("index")) -> (w1743:i32[])
            n1194 = Index Array(array=w1775, index (row) #1=w1773, index (col) #1=0, index (row) #2=w1773, index (col) #2=w1773, index (row) #3=w1773, index (col) #3=2, index (row) #4=w1773, index (col) #4=3, index (row) #5=w1773, index (col) #5=4, index (row) #6=w1773, index (col) #6=5, index (row) #7=w1773, index (col) #7=6, index (row) #8=w1773, index (col) #8=7) -> (element #1=w1766:dbl, element #2=w1765:dbl, element #3=w1764:dbl, element #4=w1763:dbl, element #5=w1762:dbl, element #6=w1761:dbl, element #7=w1760:dbl, element #8=w1759:dbl)
            n1195 = local write "estadoTorreUno"(w1743) -> ()
            n1196 = property on="PiezaUno" class="Bool (strict)"("Left"=w1766, "Top"=w1765) -> ()  [unwired: 2 in, 2 out]
            n1197 = property on="PiezaDos" class="Bool (strict)"("Left"=w1764, "Top"=w1763) -> ()  [unwired: 2 in, 2 out]
            n1198 = property on="PiezaTres" class="Bool (strict)"("Left"=w1762, "Top"=w1761) -> ()  [unwired: 2 in, 2 out]
            n1199 = property on="PiezaCuatro" class="Bool (strict)"("Left"=w1760, "Top"=w1759) -> ()  [unwired: 2 in, 2 out]
            n1200 = local write "minMov"(15.0 ("minMov")) -> ()
            n1201 = property on="PiezaUno" class="Bool (strict)"("Visible"=TRUE) -> ()  [unwired: 2 in, 2 out]
            n1202 = property on="PiezaCinco" class="Bool (strict)"("Visible"=FALSE ("PiezaCinco")) -> ()  [unwired: 2 in, 2 out]
            n1203 = property on="PiezaCuatro" class="Bool (strict)"("Visible"=TRUE ("PiezaCuatro")) -> ()  [unwired: 2 in, 2 out]
            n1204 = property on="PiezaDos" class="Bool (strict)"("Visible"=TRUE ("PiezaDos")) -> ()  [unwired: 2 in, 2 out]
            n1205 = property on="PiezaTres" class="Bool (strict)"("Visible"=TRUE) -> ()  [unwired: 2 in, 2 out]
            n1206 = property on="PiezaCinco" class="Bool (strict)"("Position"=T1 {"Left"=967, "Top"=119}) -> ()  [unwired: 2 in, 2 out]
          }
          frame "5" {
            w1803 = 2
            n1207 = local read "matrizPosIniciales"() -> (w1816:T2)
            n1208 = local write "minMov"(31.0 ("minMov")) -> ()
            n1209 = Index Array(array=w1816, index (row) #1=w1803, index (col) #1=0, index (row) #2=w1803, index (col) #2=1, index (row) #3=w1803, index (col) #3=w1803, index (row) #4=w1803, index (col) #4=3, index (row) #5=w1803, index (col) #5=4, index (row) #6=w1803, index (col) #6=5, index (row) #7=w1803, index (col) #7=6, index (row) #8=w1803, index (col) #8=7, index (row) #9=w1803, index (col) #9=8, index (row) #10=w1803, index (col) #10=9) -> (element #1=w1806:dbl, element #2=w1805:dbl, element #3=w1804:dbl, element #4=w1802:dbl, element #5=w1801:dbl, element #6=w1800:dbl, element #7=w1799:dbl, element #8=w1798:dbl, element #9=w1797:dbl, element #10=w1796:dbl)
            n1210 = property on="PiezaCinco" class="Bool (strict)"("Left"=w1797, "Top"=w1796) -> ()  [unwired: 2 in, 2 out]
            n1211 = property on="PiezaUno" class="Bool (strict)"("Left"=w1806, "Top"=w1805) -> ()  [unwired: 2 in, 2 out]
            n1212 = property on="PiezaTres" class="Bool (strict)"("Left"=w1801, "Top"=w1800) -> ()  [unwired: 2 in, 2 out]
            n1213 = property on="PiezaCuatro" class="Bool (strict)"("Left"=w1799, "Top"=w1798) -> ()  [unwired: 2 in, 2 out]
            n1214 = property on="PiezaDos" class="Bool (strict)"("Left"=w1804, "Top"=w1802) -> ()  [unwired: 2 in, 2 out]
            n1215 = Initialize Array(0, 5 ("dimension size")) -> (w1790:i32[])
            n1216 = local write "estadoTorreDos"(w1790) -> ()
            n1217 = local write "estadoTorreTres"(w1790) -> ()
            n1218 = property on="PiezaCinco" class="Bool (strict)"("Visible"=TRUE ("PiezaCinco")) -> ()  [unwired: 2 in, 2 out]
            n1219 = property on="PiezaCuatro" class="Bool (strict)"("Visible"=TRUE ("PiezaCuatro")) -> ()  [unwired: 2 in, 2 out]
            n1220 = property on="PiezaDos" class="Bool (strict)"("Visible"=TRUE ("PiezaDos")) -> ()  [unwired: 2 in, 2 out]
            n1221 = property on="PiezaTres" class="Bool (strict)"("Visible"=TRUE) -> ()  [unwired: 2 in, 2 out]
            n1222 = property on="PiezaUno" class="Bool (strict)"("Visible"=TRUE) -> ()  [unwired: 2 in, 2 out]
            n1223 = Replace Array Subset(array=w1790, new element #1=5 ("new element/subarray"), index #1=0 ("index"), new element #2=4 ("new element/subarray"), index #2=1 ("index"), new element #3=3 ("new element/subarray"), index #3=2 ("index"), new element #4=2 ("new element/subarray"), index #4=3 ("new element/subarray"), new element #5=1 ("new element/subarray"), index #5=4 ("new element/subarray")) -> (w1789:i32[])
            n1224 = local write "estadoTorreUno"(w1789) -> ()
          }
        }
        n1225 = local write "numMov"(0.0 ("minMov")) -> ()
      }
    }
  }
  "TorreUno" <- u8 100 ("TorreUno")
  "TorreDos" <- u8 100 ("TorreDos")
  "TorreTres" <- u8 100 ("TorreTres")
  "minMov" <- 0.0 ("minMov")
  "numMov" <- 0.0 ("numMov")
  "¿Pieza?" <- i8 0 ("¿Pieza?")
  "Torre" <- i8 0 ("Torre")
  "Posicion" <- 0 ("Posicion")
